vi "rio_veloster11.vi"() -> ()   [LabVIEW 2015]
uses:
  <vilib>/FPGAPlugInAG/cRIO-9113/niLvFpga_Open_cRIO-9113.vi
  <vilib>/rvi/interface/common/dynamic/niFpgaDynamicAddResources.vi
  <vilib>/FPGAPlugInAG/Dynamic/niLvFpga_Abort_Dynamic.vi
  <vilib>/FPGAPlugInAG/Dynamic/niLvFpga_Run_Dynamic.vi
  rio_Global.vi
  <vilib>/Utility/error.llb/Error Cluster From Error Code.vi
  <vilib>/rvi/errors/niLvFpgaAdjustHostInterfaceError.vi
  <vilib>/Instr/_visa.llb/VISA Configure Serial Port (Instr).vi
  <vilib>/Analysis/Matrix/Numeric/Conversions/Array To Matrix - RA2.vi
  <vilib>/Analysis/Matrix/Numeric/Multiply/Multiply - RM,RM.vi
  <vilib>/Analysis/Matrix/Numeric/Add/Add - RM,RM.vi
  <vilib>/Analysis/baseanly.llb/Real Inverse Matrix.vi
  <vilib>/Analysis/Matrix/Numeric/Subtract/Subtract - RM,RM.vi
  <vilib>/Analysis/Matrix/Numeric/Conversions/Array To Matrix - RA.vi
  <vilib>/Analysis/Matrix/Numeric/Multiply/Multiply - R,RM.vi
  <vilib>/Analysis/Matrix/Numeric/Conversions/Matrix To Array - RM.vi
  <vilib>/rvi/interface/nirviOpenFPGA/nirviOpenFPGA.xnode
  FPGA Bitfiles/autonomous_FPGATarget2_fpga4_FZHAM7r+pqE.lvbitx
  fpga/fpga4.vi
  <vilib>/rvi/interface/nirviMethod/nirviMethod.xnode
  <vilib>/rvi/interface/nirviReadWriteControl/nirviReadWriteControl.xnode
  <vilib>/Analysis/Matrix/NI_Matrix.lvlib
  <vilib>/Analysis/NI_AALBase.lvlib
  NiFpgaLv.dll
  <vilib>/rvi/interface/Simulation/niFpgaSimulationCallBeginRW.vi
panel:
  out "Heading":dbl
  out "H_GPS":dbl
  out "pos":dbl[](array[numeric])
  in  "GPS init":bool=TRUE
  out "pos_gps":dbl[](array[numeric]) format="%#_19f"
  out "dt":dbl
  out "Pos_time 10":i32
  out "battery voltage":dbl
  out "FPGA":refnum<k20>
  in  "steer limit":dbl=100.0
  in  "buzz":bool
  out "hcount":u64=1
  out "hbias":dbl
  out "vcount":u64=1
  out "vgain":dbl=1.0
  out "T PWM":u16
  out "B PWM":u16
  out "mobileye":u8[](array[numeric])
  out "timer":u32
  out "Mobileye_time 100":u32
  out "pos error":dbl
  in  "Gear Manual":i32(slide)=1 scale=-1.0..1.0
  out "map":i32=2
  out "P, R, D":i32
  out "heading error":dbl
  out "POS init":bool
  out "VS_CAN":dbl
  in  "brake":bool
  in  "Slide":dbl(slide) min=-50.0 max=50.0 step=50.0 scale=-50.0..50.0
  out "Con_time 10":i32
  out "CAN_time 10":u32
  out "ecef ref":dbl[](array[numeric])
  out "h_gps":dbl
  out "get heading":bool
  out "get position":bool
  out "rt":dbl
  out "CAN Comm Enabled":bool
  in  "SPAS Enable":bool=TRUE
  in  "file write":bool
  out "data write":refnum<file>
  out "file rw error":errorcluster
  in  "Steer input":bool=TRUE
  in  "Manual Steering angle":dbl(knob) scale=-550.0..550.0
  out "Ref vel":dbl=1.0
  in  "Manual Speed":dbl
  in  "Velocity input":bool
  out "Auto":bool
  out "Run":bool
  out "E - STOP":bool
  # "P"
  # "R"
  # "D"
  # "Manual Steering angle"
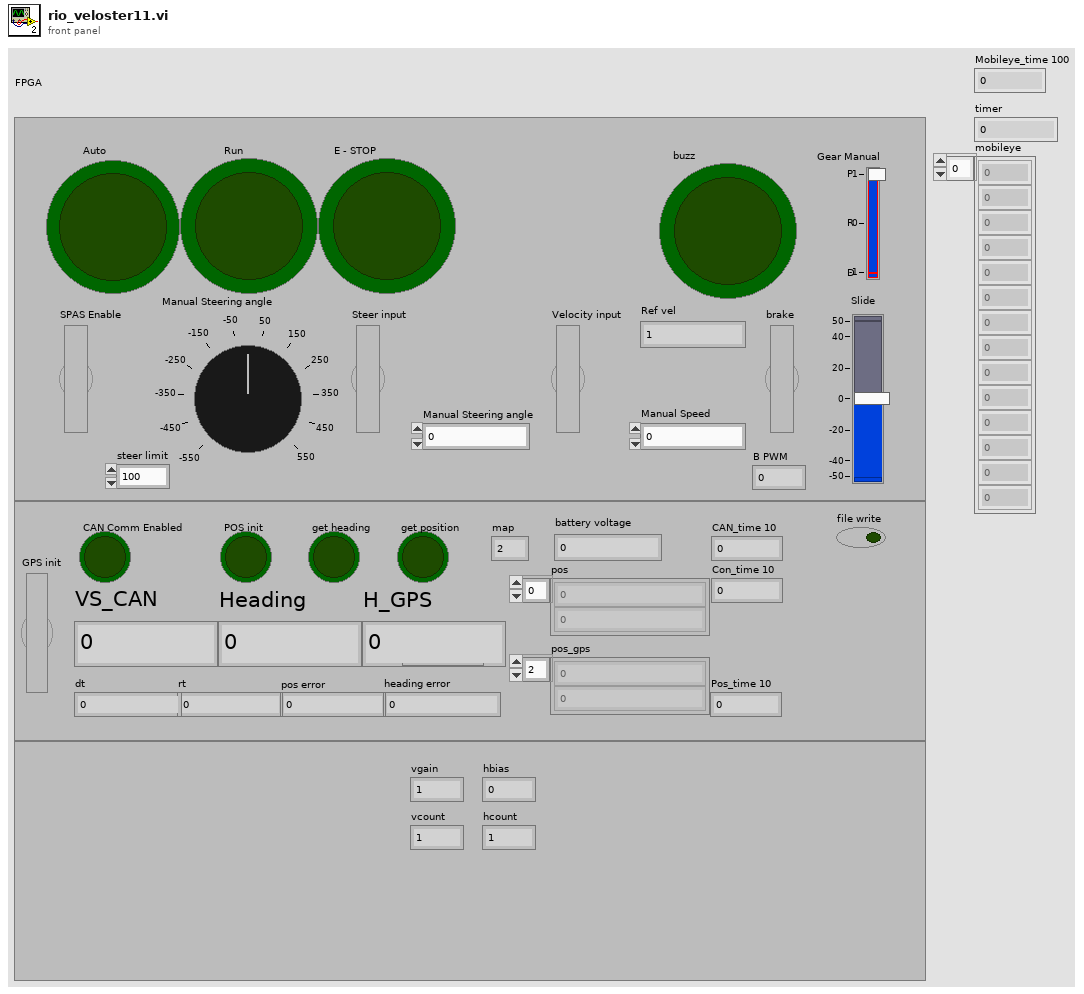
[diagram p1: front panel]
types:
  T1 = enum16{"open", "replace", "create", "open or create", "replace or create", "replace or create with confirmation"}
  T2 = cluster{"timestamp high":u32, "timestamp low":u32, "identifier":u32, "type":enum8{"Data Frame", "Remote Frame", "(reserved)", "(reserved) ", "(reserved)  ", "(reserved)   ", "Bus Error", "Transceiver Fault"}, "info A":u8, "info B":u8, "data length":u8, "data":u8[]}
  T3 = cluster{"connection ID":refnum<k16>, "net address":u32, "port":u16}
  T4 = cluster{"hash":i64, "sys time":i64, "mobileye":u8[]}
  T5 = cluster{"hash":i64, "sys time":i64, "ref_vel":dbl, "ref_steer":dbl}
  T6 = cluster{"hash":i64, "sys time":i64, "time":dbl, "yaw_rate":dbl, "mdps torque":dbl, "mdps str_ang":dbl, "VS_CAN":dbl, "lat_accel":dbl, "mcp":dbl, "accel pedal value":dbl, "tps":dbl, "odometer":dbl, "battery voltage":dbl, "WHL_SPD_RR":dbl, "WHL_SPD_RL":dbl, "WHL_SPD_FR":dbl, "WHL_SPD_FL":dbl}
  T7 = cluster{"hash":i64, "sys time":i64, "Auto":bool, "Run":bool, "Solenoid":bool, "T lim":bool, "brk_enc":u8, "B PWM":u16, "T PWM":u16, "ref_vel":dbl, "ref_bkr_enc":dbl, "ref_apv":dbl, "ref_steer":dbl}
  T8 = cluster{"hash":i64, "sys time":i64, "time":dbl, "x":dbl, "y":dbl, "h":dbl, "numSV":i32, "postype":i32, "lag":i32, "hordev":dbl, "lat":dbl, "lon":dbl, "hgt":dbl, "map_idx":i32}
  T9 = cluster{"output[0]":dbl, "output[1]":dbl, "output[2]":dbl, "output[3]":dbl, "output[4]":dbl, "output[5]":dbl, "output[6]":dbl, "output[7]":dbl, "output[8]":dbl, "output[9]":dbl, "output[10]":dbl, "output[11]":dbl, "output[12]":dbl, "output[13]":dbl, "output[14]":dbl}
  T10 = cluster{"hash":i64, "sys time":i64, "time":dbl, "speed":dbl, "heading":dbl, "lat":dbl, "lon":dbl}
  T11 = cluster{"output[0]":dbl, "output[1]":dbl, "output[2]":dbl, "output[3]":dbl, "output[4]":dbl, "output[5]":dbl, "output[6]":dbl}
  T12 = typedef "NI_Matrix.lvlib/RealMatrix.ctl" = dbl[][]
  T13 = cluster{"hash":i64, "sys time":i64, "dt":dbl, "x":dbl, "y":dbl, "speed":dbl, "heading":dbl, "yaw_rate":dbl}
  T14 = cluster{"Real 2D Array[0]":dbl, "Real 2D Array[1]":dbl, "Real 2D Array[2]":dbl, "Real 2D Array[3]":dbl, "Real 2D Array[4]":dbl}
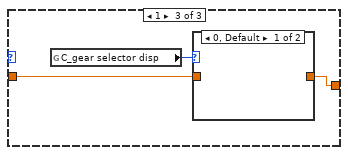
[diagram p3: hidden frame]
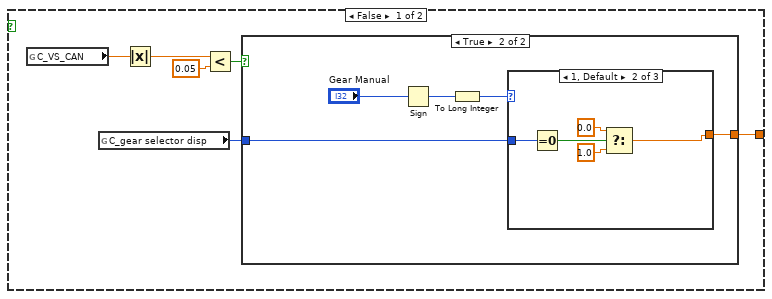
[diagram p5: hidden frame]
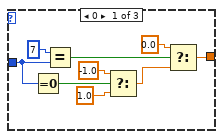
[diagram p7: hidden frame]
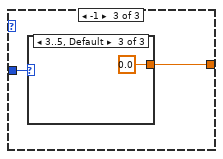
[diagram p8: hidden frame]
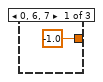
[diagram p9: hidden frame]
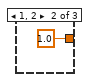
[diagram p10: hidden frame]
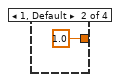
[diagram p12: hidden frame]
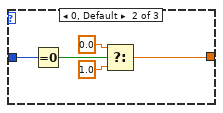
[diagram p15: hidden frame]
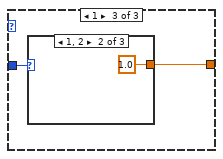
[diagram p16: hidden frame]
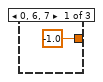
[diagram p17: hidden frame]
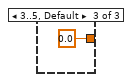
[diagram p18: hidden frame]
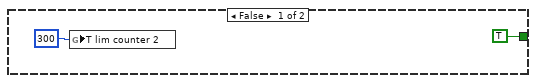
[diagram p19: hidden frame]
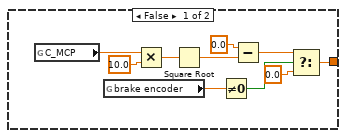
[diagram p20: hidden frame]
diagram:
  n1 = flat-sequence {
    frame #0 {
      w7 = u16 7668 ("port")
      w11 = u16 7667 ("port")
      n2 = disable-structure shown="Enabled" {
        frame Disabled {
        }
        frame Enabled {
          w21 = 0.0 ("Ref_str_ang")
          w22 = 1000.0 ("PWM GAS")
          n3 = global write "rio_Global.vi" "steering torque"(0.0 ("steering")) -> ()
          n4 = global write "rio_Global.vi" "Auto SW"(FALSE ("Auto SW")) -> ()
          n5 = global write "rio_Global.vi" "Solenoid"(FALSE ("CAN A 1")) -> ()
          n6 = global write "rio_Global.vi" "T lim counter 2"(u16 300 ("T lim counter 2")) -> ()
          n7 = global write "rio_Global.vi" "PWM GAS"(w22) -> ()
          n8 = global write "rio_Global.vi" "PWM Brake"(w22) -> ()
          n9 = global write "rio_Global.vi" "Ref_VS"(w21) -> ()
          n10 = global write "rio_Global.vi" "Ref_str_ang"(w21) -> ()
        }
      }
      n11 = xnode "Open FPGA VI Reference"() -> ("FPGA VI Reference Out"=w19:refnum<k20>, "error out"=w18:errorcluster)  [unwired: 2 in]
      n12 = global read "rio_Global.vi" "LCM PC"() -> (w3:T3)
      n13 = case shown="True" "file write" {
        frame False {
        }
        frame True {
          n14 = Open/Create/Replace File(file path (use dialog)=path "c:/datasave", operation (0:open)=T1."replace or create", access (0:read/write)=enum16{"read/write", "read-only", "write-only"}."write-only") -> (refnum out=→"data write":refnum<file>, cancelled=w29:bool, error out=→"file rw error":errorcluster)  [unwired: 3 in]
          n15 = Not(x=w29) -> (.not. x?=w28:bool)
          n16 = local write "file write"(w28) -> ()
        }
      }
      n17 = Decrement(x=w11) -> (x-1=w10:u16)
      n18 = UDP Open(11:w7) -> (port=w9:refnum<k16>)  [unwired: 4 in, 2 out]
      n19 = xnode "Invoke Method"("FPGA VI Reference In"=w19, "error in"=w18) -> ("FPGA VI Reference Out"=w17:refnum<k20>, "error out"=w16:errorcluster)
      n20 = Bundle By Name(cluster=w3, "port"=w7, "connection ID"=w9, "net address"=u32 0) -> (w4:T3)
      n21 = UDP Open(11:w10) -> (port=w13:refnum<k16>)  [unwired: 4 in, 2 out]
      n22 = xnode "Invoke Method"("FPGA VI Reference In"=w17, "error in"=w16, "Wait Until Done (F)"=FALSE) -> ("FPGA VI Reference Out"=→"FPGA":refnum<k20>)  [unwired: 1 out]
      n23 = global read "rio_Global.vi" "LCM"() -> (w6:T3)
      n24 = global write "rio_Global.vi" "LCM PC"(w4) -> ()
      n25 = Bundle By Name(cluster=w6, "port"=w11, "connection ID"=w13, "net address"=u32 4294967295) -> (w5:T3)
      n26 = global write "rio_Global.vi" "LCM"(w5) -> ()
    }
    frame #1 {
      n27 = disable-structure shown="Enabled" {
        frame Enabled {
          n28 = while {
            stop <- FALSE stop-if-true
            n29 = flat-sequence {
              frame #0 {
                n30 = Wait Until Next ms Multiple(millisecond multiple=u32 100) -> (millisecond timer value=w141:u32)
                n31 = feedback #1(w141) -> (w139:u32)
                n32 = feedback-in #1(w141) -> ()
                n33 = Subtract(x=w141, y=w139) -> (x-y=→"Mobileye_time 100":u32)
              }
              frame #1 {
                n34 = local read "FPGA"() -> (w187:refnum<k20>)
                n35 = xnode "Read/Write Control"("FPGA VI Reference In"=w187) -> ("m 700"=w147:u8[], "m 760"=w183:u8[], "m 710"=w172:u8[], "m 711"=w168:u8[], "m 720"=w166:u8[], "m 721"=w165:u8[], "m 722"=w164:u8[], "m 723"=w163:u8[], "m 724"=w162:u8[], "m 725"=w161:u8[], "m 726"=w160:u8[], "m 727"=w159:u8[], "m 728"=w158:u8[], "m 729"=w157:u8[])  [unwired: 1 in, 2 out]
                n36 = Build Array(w166, w165, w164, w163, w162, w161, w160, w159, w158, w157) -> (w156:u8[][])
                n37 = Array Subset(array=w147, index=0, length=4) -> (w144:u8[])
                n38 = Array Subset(array=w168, index=6, length=6) -> (w167:u8[])
                n39 = Index Array(array=w147, index #1=4 ("index"), index #4=8 ("index"), index #5=11 ("index")) -> (element #1=w180:u8, element #2=w179:u8, element #3=w178:u8, element #4=w177:u8, element #5=w176:u8)  [unwired: 2 in]
                n40 = Index Array(array=w144, index #1=0 ("index")) -> (element #1=w153:u8, element #2=w152:u8, element #3=w151:u8, element #4=w150:u8)  [unwired: 3 in]
                n41 = Array Subset(array=w183, index=4, length=3) -> (w175:u8[])
                n42 = Array Subset(array=w172, index=5, length=7) -> (w171:u8[])
                n43 = Build Array (concatenate)(w144, w180, w179, w178, w177, w176, w175, w171, w167) -> (w155:u8[])
                n44 = Join Numbers(hi=w153, lo=w152) -> ((hi.lo)=w149:u16)
                n45 = Join Numbers(hi=w151, lo=w150) -> ((hi.lo)=w148:u16)
                n46 = for {
                  tunnel: w156 -> [w189] mode=indexing
                  shift-right: [w192] -> w142
                  shift-left: w155 -> [w193]
                  n47 = Array Subset(array=w189, index=4, length=8) -> (w188:u8[])
                  n48 = disable-structure shown="Enabled" {
                    disable-tunnel: [w196 TRUE ("lsb carry out")] -> w194
                    disable-tunnel: w188 -> [w195 _]
                    frame Disabled {
                      n49 = Index Array(array=w195, index=0) -> (element=w198:u8)
                      n50 = Rotate Right With Carry(2:w198, 3:FALSE ("carry")) -> (1:w196:bool)  [unwired: 1 out]
                    }
                    frame Enabled {
                    }
                  }
                  n51 = case shown="True" w194 {
                    tunnel: w193 -> [w201 w204]
                    tunnel: [w201 w203] -> w192
                    tunnel: w188 -> [_ w202]
                    frame False {
                    }
                    frame True {
                      n52 = Build Array (concatenate)(w204, w202) -> (w203:u8[])
                    }
                  }
                }
                "mobileye" <- w142
                n53 = Join Numbers(hi=w149, lo=w148) -> ((hi.lo)=→"timer":u32)
              }
              frame #2 {
                n54 = Get Date/Time In Seconds() -> (seconds since 1Jan1904=w211:timestamp)
                n55 = To Double Precision Float(number=w211) -> (double precision float=w210:dbl)
                n56 = global read "rio_Global.vi" "LCM_EYE_RAW_T"() -> (w205:T4)
                n57 = Unbundle By Name(w205) -> ("hash"=w218:i64)
                n58 = Multiply(x=w210, y=1000000.0) -> (x*y=w208:dbl)
                n59 = local read "mobileye"() -> (w212:u8[])
                n60 = call "hash.vi"("input"=w218) -> ("output"=w217:i64)  [unwired: 10 in]
                n61 = To Quad Integer(1:w208) -> (0:w207:i64)
                n62 = Bundle By Name(cluster=w205, "hash"=w217, "sys time"=w207, "mobileye"=w212) -> (w216:T4)
                n63 = Flatten To String(anything=w216, prepend array or string size? (T)=FALSE) -> (data string=w215:string)  [unwired: 2 in, 2 out]
                n64 = global read "rio_Global.vi" "LCM"() -> (w206:T3)
                n65 = call "LCM_send.vi"("DATA"=w215, "ID"="EYE_RAW_T", "LCM"=w206) -> ()  [unwired: 6 in, 3 out]
              }
            }
          }
        }
        frame Disabled {
        }
      }
      n66 = while {
        stop <- FALSE stop-if-true
        n67 = global read "rio_Global.vi" "LCM PC"() -> (w128:T3)
        n68 = call "LCM_read.vi"("LCM"=w128) -> ("data"=w126:string, "ID"=w127:string)  [unwired: 7 in, 2 out]
        n69 = case shown="\"CON_INPUT_T\"" w127 {
          tunnel: w126 -> [_ w129]
          frame "False", Default {
          }
          frame "CON_INPUT_T" {
            n70 = global read "rio_Global.vi" "CON_INPUT_T"() -> (w131:T5)
            n71 = Unflatten From String(type=w131, binary string=w129, data includes array or string size? (T)=FALSE) -> (value=w130:T5, error out=w132:errorcluster)  [unwired: 2 in, 1 out]
            n72 = case shown="No Error" w132 {
              tunnel: w130 -> [w136 _]
              frame No Error {
                n73 = Unbundle By Name(w136) -> ("ref_vel"=w135:dbl, "ref_steer"=w134:dbl)
                n74 = global write "rio_Global.vi" "Ref_VS"(w135) -> ()
                n75 = global write "rio_Global.vi" "Ref_str_ang"(w134) -> ()
              }
              frame Error {
              }
            }
          }
        }
      }
      n76 = while {
        stop <- FALSE stop-if-true
        n77 = flat-sequence {
          tunnel: [w40] -> w34
          tunnel: w34 -> [w57]
          tunnel: [w56] -> w33
          tunnel: w33 -> [w111]
          frame #0 {
            n78 = Wait Until Next ms Multiple(millisecond multiple=u32 10) -> ()  [unwired: 1 out]
          }
          frame #1 {
            n79 = local read "FPGA"() -> (w42:refnum<k20>)
            n80 = xnode "Read/Write Control"("FPGA VI Reference In"=w42) -> ("FPGA VI Reference Out"=w40:refnum<k20>, "Auto"=w41:bool, "Run"=w43:bool, "T Lim"=w37:bool, "brk enc"=w53:u8)  [unwired: 1 in, 1 out]
            "Auto" <- w41
            n81 = global write "rio_Global.vi" "Auto"(w41) -> ()
            n82 = global write "rio_Global.vi" "T Lim"(w37) -> ()
            n83 = To Double Precision Float(number=w53) -> (double precision float=w45:dbl)
            n84 = And(x=w41, y=w43) -> (x .and. y?=w38:bool)
            "Run" <- w38
            n85 = global write "rio_Global.vi" "Run"(w38) -> ()
            n86 = Subtract(x=w45, y=220.0) -> (x-y=w47:dbl)
            n87 = Not(x=w38) -> (.not. x?=w55:bool)
            n88 = Multiply(x=w47, y=-100.0) -> (x*y=w50:dbl)
            n89 = And(x=w41, y=w55) -> (x .and. y?=→"E - STOP":bool)
            n90 = Divide(x=w50, y=175.0) -> (x/y=w51:dbl)
            n91 = In Range and Coerce(upper limit=100.0, x=w51, lower limit=0.0) -> (coerced(x)=w39:dbl)  [unwired: 1 out]
            n92 = global write "rio_Global.vi" "brake encoder"(w39) -> ()
          }
          frame #2 {
            n93 = global read "rio_Global.vi" "steering angle"() -> (w80:dbl)
            n94 = Multiply(x=w80, y=10.0) -> (x*y=w62:dbl)
            n95 = Greater Than 0?(x=w62) -> (x > 0?=w61:bool)
            n96 = Add(x=w62, y=65536.0) -> (x+y=w64:dbl)
            n97 = Select(t=w62, s=w61, f=w64) -> (s? t:f=w65:dbl)
            n98 = To Unsigned Word Integer(number=w65) -> (unsigned 16bit integer=w66:u16)
            n99 = Split Number(x=w66) -> (hi(x)=w67:u8, lo(x)=w68:u8)
            n100 = feedback #2(u8 0 ("Con steer alivecnt")) -> (w77:u8)
            n101 = Increment(x=w77) -> (x+1=w76:u8)
            n102 = feedback-in #2(w76) -> ()
            n103 = Build Array(u8 0 ("Con steer status"), w68, w67, u8 0 ("element"), w77, u8 0 ("element"), u8 0 ("element")) -> (w73:u8[])
            n104 = global read "rio_Global.vi" "Auto"() -> (w79:bool)
            n105 = Add Array Elements(numeric array=w73) -> (sum=w72:u8)
            n106 = And(x=w79, y="SPAS Enable") -> (x .and. y?=w58:bool)
            n107 = Build Array (concatenate)(w73, w72) -> (w78:u8[])
            n108 = case shown="True" w58 {
              tunnel: w78 -> [_ w86]
              tunnel: w57 -> [w82 w85]
              tunnel: [w81 w84] -> w56
              frame False {
                n109 = xnode "Read/Write Control"("FPGA VI Reference In"=w82, "send can"=FALSE) -> ("FPGA VI Reference Out"=w81:refnum<k20>)  [unwired: 1 in, 1 out]
              }
              frame True {
                n110 = disable-structure shown="Enabled" {
                  disable-tunnel: w86 -> [w92 _]
                  disable-tunnel: w85 -> [w88 w110]
                  disable-tunnel: [w87 w110] -> w84
                  frame Enabled {
                    n111 = flat-sequence {
                      tunnel: w92 -> [w96]
                      tunnel: [w96] -> w91
                      tunnel: [w94] -> w90
                      tunnel: w88 -> [w93]
                      tunnel: w91 -> [w101]
                      tunnel: w90 -> [w99]
                      tunnel: [w98] -> w89
                      tunnel: w89 -> [w105]
                      tunnel: [w104] -> w87
                      frame #0 {
                        n112 = xnode "Read/Write Control"("FPGA VI Reference In"=w93, "send can"=TRUE) -> ("FPGA VI Reference Out"=w94:refnum<k20>)  [unwired: 1 in, 1 out]
                      }
                      frame #1 {
                        n113 = Bundle By Name(cluster=T2 {"timestamp high"=0, "timestamp low"=0, "identifier"=0, "type"=enum."Data Frame", "info A"=0, "info B"=0, "data length"=8, "data"=[0, 0, 0, 0, 0, 0, 0, 0]} ("Mod4/CAN1 input"), "identifier"=u32 912, "data"=w101, "data length"=u8 8) -> (w100:T2)
                        n114 = xnode "Read/Write Control"("FPGA VI Reference In"=w99, "Mod4/CAN1 input"=w100) -> ("FPGA VI Reference Out"=w98:refnum<k20>)  [unwired: 1 in, 1 out]
                      }
                      frame #2 {
                        n115 = disable-structure shown="Enabled" {
                          disable-tunnel: w105 -> [w108 w109]
                          disable-tunnel: [w106 w109] -> w104
                          frame Disabled {
                            n116 = xnode "Read/Write Control"("FPGA VI Reference In"=w108, "send can"=FALSE) -> ("FPGA VI Reference Out"=w106:refnum<k20>)  [unwired: 1 in, 1 out]
                          }
                          frame Enabled {
                          }
                        }
                      }
                    }
                  }
                  frame Disabled {
                  }
                }
              }
            }
          }
          frame #3 {
            n117 = disable-structure shown="Enabled" {
              disable-tunnel: [w122 _] -> w116
              frame Enabled {
                n118 = global read "rio_Global.vi" "Auto"() -> (w121:bool)
                n119 = global read "rio_Global.vi" "Run"() -> (w120:bool)
                n120 = Compound Arithmetic op=AND(w121, w120) -> (w124:bool)
                n121 = And(x=w124, y="buzz") -> (x .and. y?=w122:bool)
              }
              frame Disabled {
              }
            }
            n122 = global read "rio_Global.vi" "PWM Brake"() -> (w114:dbl)
            n123 = global read "rio_Global.vi" "PWM GAS"() -> (w113:dbl)
            n124 = global read "rio_Global.vi" "PWM Shift"() -> (w119:dbl)
            n125 = To Unsigned Word Integer(number=w114) -> (unsigned 16bit integer=w118:u16)
            "B PWM" <- w118
            n126 = To Unsigned Word Integer(number=w113) -> (unsigned 16bit integer=w115:u16)
            "T PWM" <- w115
            n127 = global read "rio_Global.vi" "Solenoid"() -> (w112:bool)
            n128 = To Unsigned Word Integer(number=w119) -> (unsigned 16bit integer=w117:u16)
            n129 = xnode "Read/Write Control"("FPGA VI Reference In"=w111, "Buzz"=w116, "S Pwm 1"=w117, "S Pwm 2"=w117, "B Pwm"=w118, "T Pwm"=w115, "Solenoid"=w112) -> ()  [unwired: 1 in, 2 out]
          }
        }
      }
      n130 = while {
        stop <- FALSE stop-if-true
        n131 = flat-sequence {
          frame #0 {
            n132 = Wait Until Next ms Multiple(millisecond multiple=u32 10) -> (millisecond timer value=w222:u32)
            n133 = feedback #3(w222) -> (w221:u32)
            n134 = feedback-in #3(w222) -> ()
            n135 = Subtract(x=w222, y=w221) -> (x-y=→"CAN_time 10":u32)
          }
          frame #1 {
            n136 = disable-structure shown="Enabled" {
              disable-tunnel: [w225 _] -> w224
              frame Enabled {
                n137 = for {
                  tunnel: u32[] [356, 544, 809, 914, 1087, 1200, 1264, 1349] -> [w229] mode=indexing
                  tunnel: [w228] -> w226 mode=indexing
                  n138 = case shown="43F" w229 {
                    tunnel: [_ w230 w305 w344 w403 w427 w498 w530] -> w228
                    frame 0, Default {
                    }
                    frame 544 {
                      n139 = flat-sequence {
                        tunnel: [w237] -> w230
                        tunnel: [w236] -> w231
                        frame #0 {
                          n140 = local read "FPGA"() -> (w242:refnum<k20>)
                          n141 = xnode "Read/Write Control"("FPGA VI Reference In"=w242) -> ("can 220"=w241:u8[])  [unwired: 1 in, 2 out]
                          n142 = Index Array(array=w241, index #1=0 ("index")) -> (element #1=w248:u8, element #2=w247:u8, element #3=w246:u8, element #4=w245:u8)  [unwired: 3 in]
                          n143 = Join Numbers(hi=w248, lo=w247) -> ((hi.lo)=w244:u16)
                          n144 = Join Numbers(hi=w246, lo=w245) -> ((hi.lo)=w243:u16)
                          n145 = Join Numbers(hi=w244, lo=w243) -> ((hi.lo)=w234:u32)
                          n146 = Array Subset(array=w241, index=4) -> (w236:u8[])  [unwired: 1 in]
                          n147 = global write "rio_Global.vi" "C_time"(w234) -> ()
                          n148 = feedback #4(u32 0) -> (w238:u32)
                          n149 = feedback-in #4(w234) -> ()
                          n150 = Multiply(x=w234, y=1e-07) -> (x*y=w232:dbl)
                          n151 = Not Equal?(x=w234, y=w238) -> (x != y?=w237:bool)
                          n152 = feedback-in #5(w232) -> ()
                          n153 = feedback #5(w232) -> (w233:dbl)
                          n154 = global write "rio_Global.vi" "C_ts"(w233) -> ()
                        }
                      }
                      n155 = case shown="True" w230 {
                        tunnel: w231 -> [_ w283]
                        frame False {
                        }
                        frame True {
                          w253 = u16 8191
                          w260 = u16 2047
                          n156 = Index Array(array=w283, index #1=5 ("index"), index #2=4 ("index"), index #3=1 ("index"), index #4=0 ("index"), index #5=7 ("index"), index #6=6 ("index")) -> (element #1=w276:u8, element #2=w275:u8, element #3=w274:u8, element #4=w273:u8, element #5=w272:u8, element #6=w271:u8)
                          n157 = Join Numbers(hi=w274, lo=w273) -> ((hi.lo)=w261:u16)
                          n158 = Join Numbers(hi=w272, lo=w271) -> ((hi.lo)=w252:u16)
                          n159 = And(x=w276, y=u8 15) -> (x .and. y?=w269:u8)
                          n160 = Logical Shift(y=i16 -6, x=w274) -> (x << y=w263:u8)
                          n161 = Logical Shift(y=i16 -6, x=w272) -> (x << y=w256:u8)
                          n162 = Join Numbers(hi=w269, lo=w275) -> ((hi.lo)=w266:u16)
                          n163 = Equal To 0?(x=w263) -> (x = 0?=w264:bool)
                          n164 = And(x=w260, y=w261) -> (x .and. y?=w259:u16)
                          n165 = And(x=w253, y=w252) -> (x .and. y?=w251:u16)
                          n166 = Not Equal?(x=w260, y=w259) -> (x != y?=w265:bool)
                          n167 = Not Equal?(x=w253, y=w251) -> (x != y?=w254:bool)
                          n168 = Equal To 0?(x=w256) -> (x = 0?=w255:bool)
                          n169 = Not Equal?(x=u16 4095, y=w266) -> (x != y?=w267:bool)
                          n170 = case shown="True" w267 {
                            tunnel: w266 -> [_ w303]
                            frame False {
                            }
                            frame True {
                              n171 = global write "rio_Global.vi" "C_MCP"(w303) -> ()
                              n172 = Greater?(x=w303, y=u16 10) -> (0:w302:bool)
                              n173 = global write "rio_Global.vi" "C_Brake"(w302) -> ()
                            }
                          }
                          n174 = And(x=w264, y=w265) -> (x .and. y?=w258:bool)
                          n175 = And(x=w255, y=w254) -> (x .and. y?=w250:bool)
                          n176 = case shown="True" w258 {
                            tunnel: w259 -> [_ w301]
                            frame False {
                            }
                            frame True {
                              n177 = To Double Precision Float(number=w301) -> (double precision float=w300:dbl)
                              n178 = Multiply(x=w300, y=0.01) -> (x*y=w298:dbl)
                              n179 = Subtract(x=w298, y=10.23) -> (x-y=w296:dbl)
                              n180 = global write "rio_Global.vi" "C_lat_accel"(w296) -> ()
                            }
                          }
                          n181 = case shown="True" w250 {
                            tunnel: w251 -> [_ w295]
                            frame False {
                            }
                            frame True {
                              n182 = To Double Precision Float(number=w295) -> (double precision float=w294:dbl)
                              n183 = Multiply(x=w294, y=0.01) -> (x*y=w292:dbl)
                              n184 = Subtract(x=w292, y=40.95) -> (x-y=w286:dbl)
                              n185 = Add(x=w286, y=-0.034) -> (x+y=w285:dbl)
                              n186 = Multiply(x=w285, y=1.045) -> (x*y=w288:dbl)
                              n187 = Add(x=w288, y=0.0) -> (x+y=w284:dbl)
                              n188 = global write "rio_Global.vi" "C_yaw_rate"(w284) -> ()
                            }
                          }
                        }
                      }
                    }
                    frame 809 {
                      n189 = flat-sequence {
                        tunnel: [w308] -> w305
                        tunnel: [w307] -> w306
                        frame #0 {
                          n190 = local read "FPGA"() -> (w314:refnum<k20>)
                          n191 = xnode "Read/Write Control"("FPGA VI Reference In"=w314) -> ("can 329"=w313:u8[])  [unwired: 1 in, 2 out]
                          n192 = Index Array(array=w313, index #1=0 ("index")) -> (element #1=w320:u8, element #2=w319:u8, element #3=w318:u8, element #4=w317:u8)  [unwired: 3 in]
                          n193 = Join Numbers(hi=w320, lo=w319) -> ((hi.lo)=w316:u16)
                          n194 = Join Numbers(hi=w318, lo=w317) -> ((hi.lo)=w315:u16)
                          n195 = Join Numbers(hi=w316, lo=w315) -> ((hi.lo)=w309:u32)
                          n196 = Array Subset(array=w313, index=4) -> (w307:u8[])  [unwired: 1 in]
                          n197 = feedback #6(u32 0) -> (w310:u32)
                          n198 = feedback-in #6(w309) -> ()
                          n199 = Not Equal?(x=w309, y=w310) -> (x != y?=w308:bool)
                        }
                      }
                      n200 = case shown="True" w305 {
                        tunnel: w306 -> [_ w331]
                        frame False {
                        }
                        frame True {
                          # "10ms"
                          n201 = Index Array(array=w331, index #1=5 ("index"), index #2=6 ("index"), index #3=4 ("index")) -> (element #1=w328:u8, element #2=w325:u8)  [unwired: 1 out]
                          n202 = Not Equal?(x=w328, y=u8 255 ("x")) -> (x != y?=w324:bool)
                          n203 = Not Equal?(x=w325, y=u8 255 ("x")) -> (x != y?=w323:bool)
                          n204 = case shown="True" w324 {
                            tunnel: w328 -> [_ w343]
                            frame False {
                            }
                            frame True {
                              n205 = Subtract(x=w343, y=u8 32) -> (x-y=w341:u8)
                              n206 = To Double Precision Float(number=w341) -> (double precision float=w340:dbl)
                              n207 = Multiply(x=w340, y=100.0) -> (x*y=w338:dbl)
                              n208 = Divide(x=w338, y=213.0) -> (x/y=w336:dbl)
                              n209 = global write "rio_Global.vi" "C_tps"(w336) -> ()
                            }
                          }
                          n210 = case shown="True" w323 {
                            tunnel: w325 -> [_ w335]
                            frame False {
                            }
                            frame True {
                              n211 = To Double Precision Float(number=w335) -> (double precision float=w334:dbl)
                              n212 = Multiply(x=w334, y=0.3906) -> (x*y=w332:dbl)
                              n213 = global write "rio_Global.vi" "C_APV"(w332) -> ()
                            }
                          }
                        }
                      }
                    }
                    frame 914 {
                      n214 = flat-sequence {
                        tunnel: [w347] -> w344
                        tunnel: [w346] -> w345
                        frame #0 {
                          n215 = local read "FPGA"() -> (w353:refnum<k20>)
                          n216 = xnode "Read/Write Control"("FPGA VI Reference In"=w353) -> ("can 392"=w352:u8[])  [unwired: 1 in, 2 out]
                          n217 = Index Array(array=w352, index #1=0 ("index")) -> (element #1=w359:u8, element #2=w358:u8, element #3=w357:u8, element #4=w356:u8)  [unwired: 3 in]
                          n218 = Join Numbers(hi=w359, lo=w358) -> ((hi.lo)=w355:u16)
                          n219 = Join Numbers(hi=w357, lo=w356) -> ((hi.lo)=w354:u16)
                          n220 = Join Numbers(hi=w355, lo=w354) -> ((hi.lo)=w348:u32)
                          n221 = Array Subset(array=w352, index=4) -> (w346:u8[])  [unwired: 1 in]
                          n222 = feedback #7(u32 0) -> (w349:u32)
                          n223 = feedback-in #7(w348) -> ()
                          n224 = Not Equal?(x=w348, y=w349) -> (x != y?=w347:bool)
                        }
                      }
                      n225 = case shown="True" w344 {
                        tunnel: w345 -> [_ w367]
                        frame False {
                        }
                        frame True {
                          # "20ms"
                          n226 = Array Subset(array=w367, index=0, length=7) -> (w364:u8[])
                          n227 = Index Array(array=w367, index #1=7 ("index"), index #2=2 ("index"), index #3=1 ("index"), index #4=4 ("index"), index #5=3 ("index")) -> (element #1=w361:u8, element #2=w373:u8, element #3=w372:u8, element #4=w369:u8, element #5=w368:u8)
                          n228 = Add Array Elements(numeric array=w364) -> (sum=w362:u8)
                          n229 = Equal?(x=w362, y=w361) -> (x = y?=w363:bool)
                          n230 = case shown="True" w363 {
                            tunnel: w373 -> [_ w387]
                            tunnel: w372 -> [_ w386]
                            tunnel: w369 -> [_ w383]
                            tunnel: w368 -> [_ w382]
                            frame False {
                            }
                            frame True {
                              w378 = u16 4095 ("y")
                              n231 = Join Numbers(hi=w387, lo=w386) -> ((hi.lo)=w379:u16)
                              n232 = Join Numbers(hi=w383, lo=w382) -> ((hi.lo)=w384:u16)
                              n233 = And(x=w378, y=w379) -> (x .and. y?=w377:u16)
                              n234 = Not Equal?(x=w384, y=u16 32767 ("x")) -> (x != y?=w380:bool)
                              n235 = Not Equal?(x=w378, y=w377) -> (x != y?=w381:bool)
                              n236 = case shown="True" w381 {
                                tunnel: w377 -> [_ w400]
                                frame False {
                                }
                                frame True {
                                n237 = To Double Precision Float(number=w400) -> (double precision float=w399:dbl)
                                n238 = Subtract(x=w399, y=2048.0) -> (x-y=w398:dbl)
                                n239 = Multiply(x=w398, y=0.01) -> (x*y=w397:dbl)
                                n240 = global write "rio_Global.vi" "C_mdps torque"(w397) -> ()
                                }
                              }
                              n241 = case shown="True" w380 {
                                tunnel: w384 -> [_ w394]
                                frame False {
                                }
                                frame True {
                                n242 = To Double Precision Float(number=w394) -> (double precision float=w391:dbl)
                                n243 = Subtract(x=w391, y=65536.0) -> (x-y=w392:dbl)
                                n244 = Greater?(x=w391, y=32767.0 ("x")) -> (0:w395:bool)
                                n245 = Select(t=w392, s=w395, f=w391) -> (s? t:f=w390:dbl)
                                n246 = Multiply(x=w390, y=0.1) -> (x*y=w388:dbl)
                                n247 = global write "rio_Global.vi" "C_mdps str_ang"(w388) -> ()
                                }
                              }
                            }
                          }
                        }
                      }
                    }
                    frame 1087 {
                      n248 = flat-sequence {
                        tunnel: [w406] -> w403
                        tunnel: [w405] -> w404
                        frame #0 {
                          n249 = local read "FPGA"() -> (w412:refnum<k20>)
                          n250 = xnode "Read/Write Control"("FPGA VI Reference In"=w412) -> ("can 43F"=w411:u8[])  [unwired: 1 in, 2 out]
                          n251 = Index Array(array=w411, index #1=0 ("index")) -> (element #1=w418:u8, element #2=w417:u8, element #3=w416:u8, element #4=w415:u8)  [unwired: 3 in]
                          n252 = Join Numbers(hi=w418, lo=w417) -> ((hi.lo)=w414:u16)
                          n253 = Join Numbers(hi=w416, lo=w415) -> ((hi.lo)=w413:u16)
                          n254 = Join Numbers(hi=w414, lo=w413) -> ((hi.lo)=w407:u32)
                          n255 = Array Subset(array=w411, index=4) -> (w405:u8[])  [unwired: 1 in]
                          n256 = feedback #8(u32 0) -> (w408:u32)
                          n257 = feedback-in #8(w407) -> ()
                          n258 = Not Equal?(x=w407, y=w408) -> (x != y?=w406:bool)
                        }
                      }
                      n259 = case shown="True" w403 {
                        tunnel: w404 -> [_ w425]
                        frame False {
                        }
                        frame True {
                          w422 = u8 15 ("y")
                          # "10ms"
                          n260 = Index Array(array=w425, index=1) -> (element=w423:u8)
                          n261 = And(x=w423, y=w422) -> (x .and. y?=w421:u8)
                          n262 = Not Equal?(x=w421, y=w422) -> (x != y?=w420:bool)
                          n263 = case shown="True" w420 {
                            tunnel: w421 -> [_ w426]
                            frame False {
                            }
                            frame True {
                              n264 = global write "rio_Global.vi" "C_gear selector disp"(w426) -> ()
                            }
                          }
                        }
                      }
                    }
                    frame 1200 {
                      n265 = flat-sequence {
                        tunnel: [w430] -> w427
                        tunnel: [w429] -> w428
                        frame #0 {
                          n266 = local read "FPGA"() -> (w436:refnum<k20>)
                          n267 = xnode "Read/Write Control"("FPGA VI Reference In"=w436) -> ("can 4B0"=w435:u8[])  [unwired: 1 in, 2 out]
                          n268 = Index Array(array=w435, index #1=0 ("index")) -> (element #1=w442:u8, element #2=w441:u8, element #3=w440:u8, element #4=w439:u8)  [unwired: 3 in]
                          n269 = Join Numbers(hi=w442, lo=w441) -> ((hi.lo)=w438:u16)
                          n270 = Join Numbers(hi=w440, lo=w439) -> ((hi.lo)=w437:u16)
                          n271 = Join Numbers(hi=w438, lo=w437) -> ((hi.lo)=w431:u32)
                          n272 = Array Subset(array=w435, index=4) -> (w429:u8[])  [unwired: 1 in]
                          n273 = feedback #9(u32 0) -> (w432:u32)
                          n274 = feedback-in #9(w431) -> ()
                          n275 = Not Equal?(x=w431, y=w432) -> (x != y?=w430:bool)
                        }
                      }
                      n276 = case shown="True" w427 {
                        tunnel: w428 -> [_ w473]
                        frame False {
                        }
                        frame True {
                          w447 = u16 16383 ("x")
                          w460 = u16 16383 ("x")
                          # "20ms"
                          n277 = Index Array(array=w473, index #1=1 ("index"), index #2=0 ("index"), index #3=3 ("index"), index #4=2 ("index"), index #5=5 ("index"), index #6=4 ("index"), index #7=7 ("index"), index #8=6 ("index")) -> (element #1=w452:u8, element #2=w451:u8, element #3=w450:u8, element #4=w449:u8, element #5=w470:u8, element #6=w469:u8, element #7=w465:u8, element #8=w464:u8)
                          n278 = Join Numbers(hi=w452, lo=w451) -> ((hi.lo)=w448:u16)
                          n279 = Join Numbers(hi=w450, lo=w449) -> ((hi.lo)=w446:u16)
                          n280 = Join Numbers(hi=w470, lo=w469) -> ((hi.lo)=w468:u16)
                          n281 = Join Numbers(hi=w465, lo=w464) -> ((hi.lo)=w461:u16)
                          n282 = And(x=w448, y=w447) -> (x .and. y?=w445:u16)
                          n283 = And(x=w447, y=w446) -> (x .and. y?=w444:u16)
                          n284 = And(x=w468, y=w460) -> (x .and. y?=w459:u16)
                          n285 = And(x=w460, y=w461) -> (x .and. y?=w458:u16)
                          n286 = Not Equal?(x=w459, y=w460) -> (x != y?=w463:bool)
                          n287 = Not Equal?(x=w460, y=w458) -> (x != y?=w462:bool)
                          n288 = And(x=w463, y=w462) -> (x .and. y?=w457:bool)
                          n289 = case shown="True" w457 {
                            tunnel: w459 -> [_ w497]
                            tunnel: w458 -> [_ w496]
                            tunnel: w445 -> [_ w490]
                            tunnel: w444 -> [_ w489]
                            frame False {
                            }
                            frame True {
                              w486 = 0.03125 ("y")
                              w495 = 0.03125 ("y")
                              n290 = To Double Precision Float(number=w490) -> (double precision float=w487:dbl)
                              n291 = To Double Precision Float(number=w489) -> (double precision float=w485:dbl)
                              n292 = To Double Precision Float(number=w497) -> (double precision float=w488:dbl)
                              n293 = To Double Precision Float(number=w496) -> (double precision float=w484:dbl)
                              n294 = Multiply(x=w487, y=w486) -> (x*y=w483:dbl)
                              n295 = Multiply(x=w486, y=w485) -> (x*y=w482:dbl)
                              n296 = Multiply(x=w488, y=w495) -> (x*y=w481:dbl)
                              n297 = Multiply(x=w495, y=w484) -> (x*y=w480:dbl)
                              n298 = global write "rio_Global.vi" "C_WHL_SPD_FL"(w483) -> ()
                              n299 = global write "rio_Global.vi" "C_WHL_SPD_FR"(w482) -> ()
                              n300 = global write "rio_Global.vi" "C_WHL_SPD_RL"(w481) -> ()
                              n301 = global write "rio_Global.vi" "C_WHL_SPD_RR"(w480) -> ()
                              n302 = Add(x=w481, y=w480) -> (x+y=w494:dbl)
                              n303 = Multiply(x=w494, y=0.5) -> (x*y=w491:dbl)
                              n304 = global read "rio_Global.vi" "C_gear selector disp"() -> (w478:u8)
                              n305 = Multiply(x=w491, y=1.028) -> (x*y=w476:dbl)
                              n306 = Negate(x=w476) -> (-x=w477:dbl)
                              n307 = Equal?(x=w478, y=u8 7) -> (x = y?=w475:bool)
                              n308 = Select(t=w477, s=w475, f=w476) -> (s? t:f=w474:dbl)
                              n309 = global write "rio_Global.vi" "C_VS_CAN"(w474) -> ()
                            }
                          }
                        }
                      }
                    }
                    frame 1264 {
                      n310 = flat-sequence {
                        tunnel: [w501] -> w498
                        tunnel: [w500] -> w499
                        frame #0 {
                          n311 = local read "FPGA"() -> (w507:refnum<k20>)
                          n312 = xnode "Read/Write Control"("FPGA VI Reference In"=w507) -> ("can 4F0"=w506:u8[])  [unwired: 1 in, 2 out]
                          n313 = Index Array(array=w506, index #1=0 ("index")) -> (element #1=w513:u8, element #2=w512:u8, element #3=w511:u8, element #4=w510:u8)  [unwired: 3 in]
                          n314 = Join Numbers(hi=w513, lo=w512) -> ((hi.lo)=w509:u16)
                          n315 = Join Numbers(hi=w511, lo=w510) -> ((hi.lo)=w508:u16)
                          n316 = Join Numbers(hi=w509, lo=w508) -> ((hi.lo)=w502:u32)
                          n317 = Array Subset(array=w506, index=4) -> (w500:u8[])  [unwired: 1 in]
                          n318 = feedback #10(u32 0) -> (w503:u32)
                          n319 = feedback-in #10(w502) -> ()
                          n320 = Not Equal?(x=w502, y=w503) -> (x != y?=w501:bool)
                        }
                      }
                      n321 = case shown="True" w498 {
                        tunnel: w499 -> [_ w527]
                        frame False {
                        }
                        frame True {
                          # "20 ms"
                          n322 = Index Array(array=w527, index #1=7 ("index"), index #2=6 ("index"), index #3=5 ("index")) -> (element #1=w521:u8, element #2=w523:u8, element #3=w522:u8)
                          n323 = Join Numbers(hi=w523, lo=w522) -> ((hi.lo)=w518:u16)
                          n324 = Join Numbers(hi=u8 0, lo=w521) -> ((hi.lo)=w519:u16)
                          n325 = Join Numbers(hi=w519, lo=w518) -> ((hi.lo)=w516:u32)
                          n326 = Not Equal?(x=u32 16777215, y=w516) -> (x != y?=w515:bool)
                          n327 = case shown="True" w515 {
                            tunnel: w516 -> [_ w529]
                            frame False {
                            }
                            frame True {
                              n328 = To Double Precision Float(number=w529) -> (double precision float=w528:dbl)
                              n329 = global write "rio_Global.vi" "C_odometer"(w528) -> ()
                            }
                          }
                        }
                      }
                    }
                    frame 1349 {
                      n330 = flat-sequence {
                        tunnel: [w533] -> w530
                        tunnel: [w532] -> w531
                        frame #0 {
                          n331 = local read "FPGA"() -> (w539:refnum<k20>)
                          n332 = xnode "Read/Write Control"("FPGA VI Reference In"=w539) -> ("can 545"=w538:u8[])  [unwired: 1 in, 2 out]
                          n333 = Index Array(array=w538, index #1=0 ("index")) -> (element #1=w545:u8, element #2=w544:u8, element #3=w543:u8, element #4=w542:u8)  [unwired: 3 in]
                          n334 = Join Numbers(hi=w545, lo=w544) -> ((hi.lo)=w541:u16)
                          n335 = Join Numbers(hi=w543, lo=w542) -> ((hi.lo)=w540:u16)
                          n336 = Join Numbers(hi=w541, lo=w540) -> ((hi.lo)=w534:u32)
                          n337 = Array Subset(array=w538, index=4) -> (w532:u8[])  [unwired: 1 in]
                          n338 = feedback #11(u32 0) -> (w535:u32)
                          n339 = feedback-in #11(w534) -> ()
                          n340 = Not Equal?(x=w534, y=w535) -> (x != y?=w533:bool)
                        }
                      }
                      n341 = case shown="True" w530 {
                        tunnel: w531 -> [_ w547]
                        frame False {
                        }
                        frame True {
                          n342 = Index Array(array=w547, index=3) -> (element=w549:u8)
                          n343 = Not Equal?(x=w549, y=u8 255 ("x")) -> (x != y?=w551:bool)
                          n344 = case shown="True" w551 {
                            tunnel: w549 -> [_ w557]
                            frame False {
                            }
                            frame True {
                              n345 = To Double Precision Float(number=w557) -> (double precision float=w556:dbl)
                              n346 = Multiply(x=26.0, y=w556) -> (x*y=w554:dbl)
                              n347 = Divide(x=w554, y=256.0) -> (x/y=w552:dbl)
                              "battery voltage" <- w552
                              n348 = global write "rio_Global.vi" "C_battery voltage"(w552) -> ()
                            }
                          }
                        }
                      }
                    }
                  }
                }
                n349 = Or Array Elements(Boolean array=w226) -> (logical OR=w225:bool)
              }
              frame Disabled {
              }
            }
            "CAN Comm Enabled" <- w224
          }
          frame #2 {
            n350 = global read "rio_Global.vi" "C_VS_CAN"() -> (→"VS_CAN":dbl)
          }
          frame #3 {
            n351 = local read "CAN Comm Enabled"() -> (w559:bool)
            n352 = case shown="True" w559 {
              frame False {
              }
              frame True {
                n353 = Get Date/Time In Seconds() -> (seconds since 1Jan1904=w582:timestamp)
                n354 = global read "rio_Global.vi" "LCM_CAN_T"() -> (w562:T6)
                n355 = To Double Precision Float(number=w582) -> (double precision float=w581:dbl)
                n356 = global read "rio_Global.vi" "C_time"() -> (w577:u32)
                n357 = global read "rio_Global.vi" "C_battery voltage"() -> (w567:dbl)
                n358 = global read "rio_Global.vi" "C_mdps str_ang"() -> (w574:dbl)
                n359 = global read "rio_Global.vi" "C_WHL_SPD_RR"() -> (w566:dbl)
                n360 = global read "rio_Global.vi" "C_WHL_SPD_RL"() -> (w565:dbl)
                n361 = global read "rio_Global.vi" "C_WHL_SPD_FR"() -> (w564:dbl)
                n362 = global read "rio_Global.vi" "C_WHL_SPD_FL"() -> (w563:dbl)
                n363 = global read "rio_Global.vi" "C_mdps torque"() -> (w575:dbl)
                n364 = Unbundle By Name(w562) -> ("hash"=w588:i64)
                n365 = Multiply(x=w581, y=1000000.0) -> (x*y=w579:dbl)
                n366 = global read "rio_Global.vi" "C_odometer"() -> (w569:dbl)
                n367 = global read "rio_Global.vi" "C_yaw_rate"() -> (w576:dbl)
                n368 = global read "rio_Global.vi" "C_lat_accel"() -> (w572:dbl)
                n369 = global read "rio_Global.vi" "C_VS_CAN"() -> (w573:dbl)
                n370 = global read "rio_Global.vi" "C_MCP"() -> (w571:dbl)
                n371 = global read "rio_Global.vi" "C_APV"() -> (w570:dbl)
                n372 = To Quad Integer(1:w579) -> (0:w578:i64)
                n373 = call "hash.vi"("input"=w588) -> ("output"=w587:i64)  [unwired: 10 in]
                n374 = To Double Precision Float(number=w577) -> (double precision float=w586:dbl)
                n375 = global read "rio_Global.vi" "C_tps"() -> (w568:dbl)
                n376 = Bundle By Name(cluster=w562, "hash"=w587, "sys time"=w578, "time"=w586, "yaw_rate"=w576, "mdps torque"=w575, "mdps str_ang"=w574, "VS_CAN"=w573, "lat_accel"=w572, "mcp"=w571, "accel pedal value"=w570, "tps"=w568, "odometer"=w569, "battery voltage"=w567, "WHL_SPD_RR"=w566, "WHL_SPD_RL"=w565, "WHL_SPD_FR"=w564, "WHL_SPD_FL"=w563) -> (w585:T6)
                n377 = Flatten To String(anything=w585, prepend array or string size? (T)=FALSE) -> (data string=w584:string)  [unwired: 2 in, 2 out]
                n378 = global read "rio_Global.vi" "LCM"() -> (w560:T3)
                n379 = call "LCM_send.vi"("DATA"=w584, "ID"="CAN_T", "LCM"=w560) -> ()  [unwired: 6 in, 3 out]
              }
            }
          }
        }
      }
    }
  }
  n380 = flat-sequence {
    frame #0 {
      w593 = FALSE ("GPS init")
      n381 = local write "Manual Steering angle"(0.0 ("steer manual")) -> ()
      n382 = local write "Manual Speed"(0.0 ("Manual Speed")) -> ()
      n383 = local write "Steer input"(TRUE ("Steer input")) -> ()
      n384 = call "car_spec.vi"("Car_name"="Veloster") -> ()  [unwired: 11 in]
      n385 = local write "brake"(w593) -> ()
      n386 = local write "Velocity input"(w593) -> ()
    }
    frame #1 {
      n387 = while {
        stop <- FALSE stop-if-true
        n388 = flat-sequence {
          frame #0 {
            n389 = Wait Until Next ms Multiple(millisecond multiple=u32 10) -> (millisecond timer value=w598:u32)
            n390 = feedback #12(w598) -> (w597:u32)
            n391 = feedback-in #12(w598) -> ()
            n392 = Subtract(x=w598, y=w597) -> (x-y=w596:u32)
            n393 = To Long Integer(number=w596) -> (32bit integer=→"Con_time 10":i32)
          }
          frame #1 {
            n394 = flat-sequence {
              frame #0 {
                n395 = global read "rio_Global.vi" "C_mdps str_ang"() -> (w620:dbl)
                n396 = global read "rio_Global.vi" "C_mdps str_ang"() -> (w619:dbl)
                n397 = global read "rio_Global.vi" "Ref_str_ang"() -> (w618:dbl)
                n398 = Negate(x="Manual Steering angle") -> (-x=w622:dbl)
                n399 = Add(x=w620, y="steer limit") -> (x+y=w626:dbl)
                n400 = Subtract(x=w619, y="steer limit") -> (x-y=w625:dbl)
                n401 = Select(t=w618, s="Steer input", f=w622) -> (s? t:f=w624:dbl)
                n402 = In Range and Coerce(upper limit=w626, x=w624, lower limit=w625) -> (coerced(x)=w617:dbl)  [unwired: 1 out]
                n403 = global write "rio_Global.vi" "steering angle"(w617) -> ()
              }
            }
            n404 = global read "rio_Global.vi" "Ref_VS"() -> (w600:dbl)
            n405 = Select(t=w600, s="Velocity input", f="Manual Speed") -> (s? t:f=w603:dbl)
            n406 = To Long Integer(number=w603) -> (32bit integer=w602:i32)
            n407 = Sign(1:w602) -> (0:w601:i32)
            "P, R, D" <- w601
            n408 = case shown="-1" w601 {
              tunnel: [w608 _ w615] -> w604
              tunnel: w603 -> [w610 _ w614]
              frame -1 {
                n409 = global read "rio_Global.vi" "C_gear selector disp"() -> (w607:u8)
                n410 = Equal?(x=w607, y=u8 7) -> (x = y?=w611:bool)
                n411 = Select(t=w610, s=w611, f=0.0) -> (s? t:f=w608:dbl)
              }
              frame 0, Default {
              }
              frame 1 {
                n412 = global read "rio_Global.vi" "C_gear selector disp"() -> (w613:u8)
                n413 = case shown="0, Default" w613 {
                  tunnel: [_ w616] -> w615
                  tunnel: w614 -> [_ w616]
                  frame 0, Default {
                  }
                  frame 4, 5 {
                  }
                }
              }
            }
            "Ref vel" <- w604
          }
          frame #2 {
            n414 = global read "rio_Global.vi" "Auto"() -> (w636:bool)
            n415 = case shown="True" w636 {
              tunnel: [w639 w674] -> w628
              frame False {
                n416 = global read "rio_Global.vi" "C_VS_CAN"() -> (w638:dbl)
                n417 = global read "rio_Global.vi" "C_gear selector disp"() -> (w637:u8)
                n418 = Absolute Value(x=w638) -> (abs(x)=w642:dbl)
                n419 = Less?(x=w642, y=0.05) -> (x < y?=w640:bool)
                n420 = case shown="True" w640 {
                  tunnel: [_ w646] -> w639
                  tunnel: w637 -> [_ w643]
                  frame False {
                  }
                  frame True {
                    n421 = Sign(1:"Gear Manual") -> (0:w647:i32)
                    n422 = To Long Integer(number=w647) -> (32bit integer=w645:i32)
                    n423 = case shown="1, Default" w645 {
                      tunnel: [w654 w659 w663] -> w646
                      tunnel: w643 -> [w648 w657 w662]
                      frame 0 {
                        n424 = Equal To 0?(x=w648) -> (x = 0?=w652:bool)
                        n425 = Equal?(x=u8 7 ("y"), y=w648) -> (x = y?=w656:bool)
                        n426 = Select(t=-1.0, s=w652, f=1.0) -> (s? t:f=w651:dbl)
                        n427 = Select(t=0.0, s=w656, f=w651) -> (s? t:f=w654:dbl)
                      }
                      frame 1, Default {
                        n428 = Equal To 0?(x=w657) -> (x = 0?=w661:bool)
                        n429 = Select(t=0.0, s=w661, f=1.0 ("t")) -> (s? t:f=w659:dbl)
                      }
                      frame -1 {
                        n430 = case shown="3..5, Default" w662 {
                          tunnel: [-1.0 1.0 0.0] -> w663
                          frame 0, 6, 7 {
                          }
                          frame 1, 2 {
                          }
                          frame 3..5, Default {
                          }
                        }
                      }
                    }
                  }
                }
              }
              frame True {
                n431 = global read "rio_Global.vi" "C_VS_CAN"() -> (w669:dbl)
                n432 = Absolute Value(x=w669) -> (abs(x)=w672:dbl)
                n433 = global read "rio_Global.vi" "C_gear selector disp"() -> (w667:u8)
                n434 = Less?(x=w672, y=0.05) -> (x < y?=w670:bool)
                n435 = global read "rio_Global.vi" "Run"() -> (w668:bool)
                n436 = And(x=w670, y=w668) -> (x .and. y?=w673:bool)
                n437 = case shown="True" w673 {
                  tunnel: [_ w677] -> w674
                  tunnel: w667 -> [_ w675]
                  frame False {
                  }
                  frame True {
                    n438 = local read "P, R, D"() -> (w676:i32)
                    n439 = case shown="-1" w676 {
                      tunnel: [w679 w684 w688] -> w677
                      tunnel: w675 -> [w678 w682 w687]
                      frame -1 {
                        n440 = case shown="0" w678 {
                          tunnel: [-1.0 ("t") 1.0 ("t") _ _] -> w679
                          frame 0 {
                          }
                          frame 1, Default {
                          }
                          frame 4, 8 {
                          }
                          frame 7 {
                          }
                        }
                      }
                      frame 0, Default {
                        n441 = Equal To 0?(x=w682) -> (x = 0?=w686:bool)
                        n442 = Select(t=0.0, s=w686, f=1.0 ("t")) -> (s? t:f=w684:dbl)
                      }
                      frame 1 {
                        n443 = case shown="1, 2" w687 {
                          tunnel: [-1.0 1.0 0.0] -> w688
                          frame 0, 6, 7 {
                          }
                          frame 1, 2 {
                          }
                          frame 3..5, Default {
                          }
                        }
                      }
                    }
                  }
                }
              }
            }
            n444 = Multiply(x=w628, y=250.0 ("S gain")) -> (x*y=w633:dbl)
            n445 = In Range and Coerce(upper limit=500.0, x=w633, lower limit=-500.0) -> (coerced(x)=w630:dbl)  [unwired: 1 out]
            n446 = Add(x=w630, y=1500.0) -> (x+y=w635:dbl)
            n447 = global write "rio_Global.vi" "PWM Shift"(w635) -> ()
          }
          frame #3 {
            n448 = flat-sequence {
              frame #0 {
                n449 = global read "rio_Global.vi" "Auto"() -> (w692:bool)
                n450 = flat-sequence {
                  tunnel: [w703] -> w694
                  frame #0 {
                    n451 = global read "rio_Global.vi" "C_APV"() -> (w708:dbl)
                    n452 = Equal To 0?(x=w708) -> (x = 0?=w710:bool)
                    n453 = case shown="True" w710 {
                      tunnel: [TRUE w718] -> w711
                      frame False {
                        n454 = global write "rio_Global.vi" "T lim counter 2"(u16 300 ("T lim counter 2")) -> ()
                      }
                      frame True {
                        n455 = global read "rio_Global.vi" "T lim counter 2"() -> (w716:u16)
                        n456 = Decrement(x=w716) -> (x-1=w719:u16)
                        n457 = Max & Min(x=u16 0, y=w719) -> (max(x,y)=w717:u16)  [unwired: 1 out]
                        n458 = Not Equal To 0?(x=w717) -> (x != 0?=w718:bool)
                        n459 = global write "rio_Global.vi" "T lim counter 2"(w717) -> ()
                      }
                    }
                    n460 = global read "rio_Global.vi" "Throttle_Enable"() -> (w704:bool)
                    n461 = global read "rio_Global.vi" "C_Brake"() -> (w705:bool)
                    n462 = local read "Ref vel"() -> (w709:dbl)
                    n463 = Not Equal To 0?(x=w709) -> (x != 0?=w713:bool)
                    n464 = Not(x=w705) -> (.not. x?=w712:bool)
                    n465 = global read "rio_Global.vi" "Auto"() -> (w707:bool)
                    n466 = global read "rio_Global.vi" "Run"() -> (w706:bool)
                    n467 = Compound Arithmetic op=AND(w707, w706, w713, w712, w704, w711) -> (w703:bool)
                    n468 = global write "rio_Global.vi" "Solenoid"(w703) -> ()
                  }
                }
                n469 = case shown="True" w692 {
                  tunnel: [w760 w774] -> w693
                  frame False {
                    n470 = global read "rio_Global.vi" "C_MCP"() -> (w757:dbl)
                    n471 = global read "rio_Global.vi" "brake encoder"() -> (w753:dbl)
                    n472 = Multiply(x=w757, y=10.0) -> (x*y=w755:dbl)
                    n473 = Square Root(x=w755) -> (sqrt(x)=w754:dbl)
                    n474 = Not Equal To 0?(x=w753) -> (x != 0?=w759:bool)
                    n475 = Subtract(x=0.0, y=w754) -> (x-y=w761:dbl)
                    n476 = Select(t=w761, s=w759, f=0.0) -> (s? t:f=w760:dbl)
                  }
                  frame True {
                    n477 = global read "rio_Global.vi" "Run"() -> (w763:bool)
                    n478 = case shown="False" w763 {
                      tunnel: [w776 w781] -> w772
                      frame False {
                        n479 = global read "rio_Global.vi" "Const Brk FULL"() -> (w776:dbl)
                      }
                      frame True {
                        n480 = global read "rio_Global.vi" "C_VS_CAN"() -> (w777:dbl)
                        n481 = global read "rio_Global.vi" "Const Brk FULL"() -> (w780:dbl)
                        n482 = local read "Ref vel"() -> (w779:dbl)
                        n483 = Equal To 0?(x=w779) -> (x = 0?=w783:bool)
                        n484 = call "B_control.vi"("Ref vel"=w779, "VS_CAN"=w777) -> ("Ref Brk Enc"=w778:dbl)  [unwired: 17 in]
                        n485 = Select(t=w780, s=w783, f=w778) -> (s? t:f=w782:dbl)
                        n486 = Max & Min(x=w780, y=w782) -> (min(x,y)=w781:dbl)  [unwired: 1 out]
                      }
                    }
                    n487 = global read "rio_Global.vi" "C_MCP"() -> (w768:dbl)
                    n488 = global read "rio_Global.vi" "brake encoder"() -> (w764:dbl)
                    n489 = Multiply(x=w768, y=10.0) -> (x*y=w766:dbl)
                    n490 = Square Root(x=w766) -> (sqrt(x)=w765:dbl)
                    n491 = Subtract(x=w772, y=w765) -> (x-y=w773:dbl)
                    n492 = Equal To 0?(x=w764) -> (x = 0?=w770:bool)
                    n493 = Equal To 0?(x=w772) -> (x = 0?=w771:bool)
                    n494 = And(x=w770, y=w771) -> (x .and. y?=w769:bool)
                    n495 = Select(t=0.0, s=w769, f=w773) -> (s? t:f=w774:dbl)
                  }
                }
                n496 = flat-sequence {
                  tunnel: w693 -> [w748]
                  frame #0 {
                    w723 = 0.2 ("x")
                    n497 = Multiply(x=w748, y=-0.01) -> (x*y=w750:dbl)
                    n498 = In Range and Coerce(upper limit=1.0 ("x"), x=w750, lower limit=-1.0) -> (coerced(x)=w741:dbl)  [unwired: 1 out]
                    n499 = Subtract(x=1.0, y=w723) -> (x-y=w725:dbl)
                    n500 = Multiply(x=w741, y=w723) -> (x*y=w727:dbl)
                    n501 = feedback #13(0.0) -> (w724:dbl)
                    n502 = Multiply(x=w725, y=w724) -> (x*y=w726:dbl)
                    n503 = Add(x=w727, y=w726) -> (x+y=w742:dbl)
                    n504 = feedback-in #13(w742) -> ()
                    n505 = Multiply(x=w741, y=1.8 ("B P gain")) -> (x*y=w722:dbl)
                    n506 = call "deadzone.vi"("min"=-15.0, "max"=15.0, "x"=w742) -> ("dead zone"=w743:dbl)  [unwired: 8 in]
                    n507 = Multiply(x=w743, y=0.1 ("B D gain")) -> (x*y=w721:dbl)
                    n508 = Add(x=w722, y=w721) -> (x+y=w730:dbl)
                    n509 = Multiply(x=w730, y=600.0 ("B gain")) -> (x*y=w738:dbl)
                    n510 = Select(t=w738, s="brake", f="Slide") -> (s? t:f=w736:dbl)
                    n511 = In Range and Coerce(upper limit=500.0, x=w736, lower limit=-500.0) -> (coerced(x)=w735:dbl)  [unwired: 1 out]
                    n512 = Add(x=w735, y=1500.0) -> (x+y=w740:dbl)
                    n513 = global write "rio_Global.vi" "PWM Brake"(w740) -> ()
                  }
                }
                n514 = case shown="True" w694 {
                  tunnel: [w784 w827] -> w702
                  frame False {
                    n515 = flat-sequence {
                      tunnel: [w794] -> w784
                      frame #0 {
                        n516 = global read "rio_Global.vi" "T Lim"() -> (w785:bool)
                        n517 = case shown="True" w785 {
                          selector: w785 -> [_ w790]
                          frame False {
                            n518 = global write "rio_Global.vi" "T lim counter"(u16 0 ("T lim counter")) -> ()
                          }
                          frame True {
                            n519 = global write "rio_Global.vi" "T lim once"(w790) -> ()
                            n520 = global write "rio_Global.vi" "T lim counter 2"(u16 300 ("T lim counter 2")) -> ()
                            n521 = global read "rio_Global.vi" "T lim counter"() -> (w787:u16)
                            n522 = Increment(x=w787) -> (x+1=w792:u16)
                            n523 = Max & Min(x=u16 100, y=w792) -> (min(x,y)=w788:u16)  [unwired: 1 out]
                            n524 = global write "rio_Global.vi" "T lim counter"(w788) -> ()
                          }
                        }
                      }
                      frame #1 {
                        n525 = global read "rio_Global.vi" "T lim once"() -> (w793:bool)
                        n526 = case shown="True" w793 {
                          tunnel: [-1.0 ("t") w799] -> w794
                          frame False {
                          }
                          frame True {
                            n527 = global read "rio_Global.vi" "T lim counter"() -> (w796:u16)
                            n528 = Equal?(x=w796, y=u16 100) -> (x = y?=w798:bool)
                            n529 = Select(t=0.0, s=w798, f=-0.15) -> (s? t:f=w799:dbl)
                          }
                        }
                        n530 = global write "rio_Global.vi" "Throttle_Enable"(w793) -> ()
                      }
                    }
                  }
                  frame True {
                    n531 = global write "rio_Global.vi" "T lim counter"(u16 0 ("T lim counter")) -> ()
                    n532 = global write "rio_Global.vi" "T lim once"(FALSE ("T lim once")) -> ()
                    n533 = global read "rio_Global.vi" "C_VS_CAN"() -> (w807:dbl)
                    n534 = local read "Ref vel"() -> (w806:dbl)
                    n535 = global read "rio_Global.vi" "C_APV"() -> (w803:dbl)
                    n536 = call "T_control.vi"("Ref vel"=w806, "VS_CAN"=w807, "pid gain"=dbl[] [3.0, 0.0, 0.10000000000000003] ("pid gain 1")) -> ("Ref APS"=w804:dbl)  [unwired: 16 in]
                    n537 = global read "rio_Global.vi" "C_APV"() -> (w802:dbl)
                    n538 = Subtract(x=w804, y=w803) -> (x-y=w815:dbl)
                    n539 = flat-sequence {
                      tunnel: w815 -> [w848]
                      tunnel: [w845] -> w822
                      frame #0 {
                        n540 = feedback #14(0.0) -> (w853:dbl)
                        n541 = feedback-in #14(w848) -> ()
                        n542 = Multiply(x=w848, y=0.01) -> (x*y=w849:dbl)
                        n543 = Subtract(x=w848, y=w853) -> (x-y=w852:dbl)
                        n544 = feedback #15(0.0) -> (w844:dbl)
                        n545 = Multiply(x=0.999, y=w844) -> (x*y=w843:dbl)
                        n546 = Divide(x=w852, y=0.01) -> (x/y=w839:dbl)
                        n547 = Add(x=w849, y=w843) -> (x+y=w840:dbl)
                        n548 = feedback-in #15(w840) -> ()
                        n549 = Build Array(w848, w840, w839) -> (w847:dbl[])
                        n550 = Multiply(x=w847, y=dbl[] [8.0, 0.02, 0.4] ("pid gain 2")) -> (x*y=w846:dbl[])
                        n551 = Add Array Elements(numeric array=w846) -> (sum=w845:dbl)
                      }
                    }
                    n552 = Equal To 0?(x=w802) -> (x = 0?=w808:bool)
                    n553 = Greater Than 0?(x=w815) -> (x > 0?=w816:bool)
                    n554 = Less Than 0?(x=w815) -> (x < 0?=w809:bool)
                    n555 = Greater?(x=w802, y=95.0) -> (0:w817:bool)
                    n556 = And(x=w817, y=w816) -> (x .and. y?=w813:bool)
                    n557 = And(x=w808, y=w809) -> (x .and. y?=w814:bool)
                    n558 = Or(x=w813, y=w814) -> (x .or. y?=w812:bool)
                    n559 = Multiply(x=w822, y=0.01) -> (x*y=w820:dbl)
                    n560 = In Range and Coerce(upper limit=1.0 ("x"), x=w820, lower limit=-1.0) -> (coerced(x)=w811:dbl)  [unwired: 1 out]
                    n561 = flat-sequence {
                      tunnel: w811 -> [w829]
                      tunnel: [w835] -> w810
                      frame #0 {
                        w828 = 0.5 ("x")
                        n562 = Multiply(x=w829, y=w828) -> (x*y=w833:dbl)
                        n563 = Subtract(x=1.0, y=w828) -> (x-y=w831:dbl)
                        n564 = feedback #16(0.0) -> (w830:dbl)
                        n565 = Multiply(x=w831, y=w830) -> (x*y=w832:dbl)
                        n566 = Add(x=w833, y=w832) -> (x+y=w835:dbl)
                        n567 = feedback-in #16(w835) -> ()
                      }
                    }
                    n568 = Select(t=0.0 ("f"), s=w812, f=w810) -> (s? t:f=w827:dbl)
                  }
                }
                n569 = Multiply(x=w702, y=500.0 ("T gain")) -> (x*y=w700:dbl)
                n570 = In Range and Coerce(upper limit=500.0, x=w700, lower limit=-500.0) -> (coerced(x)=w696:dbl)  [unwired: 1 out]
                n571 = Add(x=w696, y=1500.0) -> (x+y=w695:dbl)
                n572 = global write "rio_Global.vi" "PWM GAS"(w695) -> ()
              }
              frame #1 {
                w858 = 0.0 ("ref_bkr_enc")
                n573 = Get Date/Time In Seconds() -> (seconds since 1Jan1904=w872:timestamp)
                n574 = global read "rio_Global.vi" "LCM_CON_T"() -> (w857:T7)
                n575 = To Double Precision Float(number=w872) -> (double precision float=w871:dbl)
                n576 = global read "rio_Global.vi" "brake encoder"() -> (w855:dbl)
                n577 = global read "rio_Global.vi" "PWM Brake"() -> (w862:dbl)
                n578 = global read "rio_Global.vi" "PWM GAS"() -> (w860:dbl)
                n579 = global read "rio_Global.vi" "steering angle"() -> (w867:dbl)
                n580 = Unbundle By Name(w857) -> ("hash"=w878:i64)
                n581 = Multiply(x=w871, y=1000000.0) -> (x*y=w869:dbl)
                n582 = global read "rio_Global.vi" "Solenoid"() -> (w866:bool)
                n583 = call "hash.vi"("input"=w878) -> ("output"=w877:i64)  [unwired: 10 in]
                n584 = To Quad Integer(1:w869) -> (0:w868:i64)
                n585 = To Unsigned Byte Integer(number=w855) -> (unsigned 8bit integer=w854:u8)
                n586 = To Unsigned Word Integer(number=w862) -> (unsigned 16bit integer=w861:u16)
                n587 = To Unsigned Word Integer(number=w860) -> (unsigned 16bit integer=w859:u16)
                n588 = local read "Ref vel"() -> (w873:dbl)
                n589 = global read "rio_Global.vi" "T Lim"() -> (w863:bool)
                n590 = global read "rio_Global.vi" "Auto"() -> (w865:bool)
                n591 = global read "rio_Global.vi" "Run"() -> (w864:bool)
                n592 = Bundle(cluster=w857, "hash"=w877, "sys time"=w868, "Auto"=w865, "Run"=w864, "Solenoid"=w866, "T lim"=w863, "brk_enc"=w854, "B PWM"=w861, "T PWM"=w859, "ref_vel"=w873, "ref_bkr_enc"=w858, "ref_apv"=w858, "ref_steer"=w867) -> (w874:T7)
                n593 = Flatten To String(anything=w874, prepend array or string size? (T)=FALSE) -> (data string=w875:string)  [unwired: 2 in, 2 out]
                n594 = global read "rio_Global.vi" "LCM"() -> (w856:T3)
                n595 = call "LCM_send.vi"("DATA"=w875, "ID"="CON_T", "LCM"=w856) -> ()  [unwired: 6 in, 3 out]
              }
            }
          }
        }
      }
    }
  }
  n596 = flat-sequence {
    tunnel: [dbl[] [0.0, 0.0, 0.0, 0.0, 0.0] ("pos(i)")] -> w1
    tunnel: w1 -> [w888]
    frame #0 {
      w884 = 10 ("map")
      w881 = FALSE ("get heading")
      w887 = u64 1
      w886 = 0.0 ("dh_hat")
      n597 = call "getecefdcmref.vi"("map"=w884) -> ("XYZ"=→"ecef ref":dbl[])  [unwired: 10 in, 4 out]
      "vgain" <- 1.0 ("initH")
      "vcount" <- w887
      "hbias" <- w886
      "hcount" <- w887
      "get heading" <- w881
      "get position" <- w881
      "heading error" <- w886
      "h_gps" <- w886
      "rt" <- w886
      "pos error" <- w886
      "map" <- w884
      "POS init" <- TRUE ("pos linit")
    }
    frame #1 {
      n598 = flat-sequence {
        frame #0 {
          n599 = call-poly "VISA Configure Serial Port"("VISA resource name"=refnum<visa-resource-name> "USB0::0x1546::0x01A6::NI-VISA-1::1::RAW", "timeout (10sec)"=u32 1, "baud rate (9600)"=u32 115200) -> ("VISA resource name out"=w964:refnum<visa-resource-name>)  [unwired: 11 in, 1 out]
          n600 = while {
            tunnel: w964 -> [w965]
            stop <- FALSE stop-if-true
            n601 = VISA Read(VISA resource name=w965, byte count=u32 100) -> (read buffer=w966:string)  [unwired: 1 in, 3 out]
            n602 = case shown="Default" w966 {
              selector: w966 -> [_ w970]
              frame "" {
                n603 = Wait (ms)(milliseconds to wait=u32 20) -> ()  [unwired: 1 out]
              }
              frame Default {
                n604 = local read "ecef ref"() -> (w971:dbl[])
                n605 = call "nmea.vi"("ecef ref"=w971, "NMEA"=w970) -> ("output"=w973:dbl[], "type"=w972:u32)  [unwired: 8 in]
                n606 = case shown="1" w972 {
                  tunnel: w973 -> [_ w975 w1008]
                  frame 0, Default {
                  }
                  frame 1 {
                    n607 = global write "rio_Global.vi" "gps_pos 1"(w975) -> ()
                    n608 = Index Array(array=w975, index=1) -> (element=w977:dbl)
                    n609 = Not Equal To 0?(x=w977) -> (x != 0?=w974:bool)
                    n610 = case shown="True" w974 {
                      tunnel: w975 -> [_ w997]
                      frame False {
                      }
                      frame True {
                        n611 = Get Date/Time In Seconds() -> (seconds since 1Jan1904=w982:timestamp)
                        n612 = To Double Precision Float(number=w982) -> (double precision float=w981:dbl)
                        n613 = global read "rio_Global.vi" "LCM_GGA_T"() -> (w1006:T8)
                        n614 = Array To Cluster(array=w997) -> (cluster=w1005:T9)
                        n615 = Unbundle By Name(w1006) -> ("hash"=w1002:i64)
                        n616 = Multiply(x=w981, y=1000000.0) -> (x*y=w979:dbl)
                        n617 = Unbundle(w1005) -> ("output[0]"=w1007:dbl, "output[2]"=w996:dbl, "output[3]"=w995:dbl, "output[4]"=w994:dbl, "output[6]"=w993:dbl, "output[7]"=w991:dbl, "output[8]"=w989:dbl, "output[9]"=w987:dbl, "output[12]"=w986:dbl, "output[13]"=w985:dbl, "output[14]"=w984:dbl)  [unwired: 4 out]
                        n618 = call "hash.vi"("input"=w1002) -> ("output"=w1001:i64)  [unwired: 10 in]
                        n619 = To Quad Integer(1:w979) -> (0:w978:i64)
                        n620 = To Long Integer(number=w993) -> (32bit integer=w992:i32)
                        n621 = To Long Integer(number=w991) -> (32bit integer=w990:i32)
                        n622 = To Long Integer(number=w989) -> (32bit integer=w988:i32)
                        n623 = local read "map"() -> (w983:i32)
                        n624 = Bundle(cluster=w1006, "hash"=w1001, "sys time"=w978, "time"=w1007, "x"=w996, "y"=w995, "h"=w994, "numSV"=w992, "postype"=w990, "lag"=w988, "hordev"=w987, "lat"=w986, "lon"=w985, "hgt"=w984, "map_idx"=w983) -> (w1003:T8)
                        n625 = Flatten To String(anything=w1003, prepend array or string size? (T)=FALSE) -> (data string=w999:string)  [unwired: 2 in, 2 out]
                        n626 = global read "rio_Global.vi" "LCM"() -> (w998:T3)
                        n627 = call "LCM_send.vi"("DATA"=w999, "ID"="GGA_1", "LCM"=w998) -> ()  [unwired: 6 in, 3 out]
                      }
                    }
                  }
                  frame 2 {
                    n628 = flat-sequence {
                      tunnel: w1008 -> [w1010]
                      frame #0 {
                        n629 = Index Array(array=w1010, index=1) -> (element=w1012:dbl)
                        n630 = Not Equal To 0?(x=w1012) -> (x != 0?=w1009:bool)
                        n631 = case shown="True" w1009 {
                          tunnel: w1010 -> [_ w1031]
                          frame False {
                          }
                          frame True {
                            n632 = Get Date/Time In Seconds() -> (seconds since 1Jan1904=w1017:timestamp)
                            n633 = To Double Precision Float(number=w1017) -> (double precision float=w1016:dbl)
                            n634 = global read "rio_Global.vi" "LCM_RMC_T"() -> (w1032:T10)
                            n635 = Unbundle By Name(w1032) -> ("hash"=w1028:i64)
                            n636 = Multiply(x=w1016, y=1000000.0) -> (x*y=w1014:dbl)
                            n637 = Array To Cluster(array=w1031) -> (cluster=w1030:T11)
                            n638 = To Quad Integer(1:w1014) -> (0:w1013:i64)
                            n639 = call "hash.vi"("input"=w1028) -> ("output"=w1027:i64)  [unwired: 10 in]
                            n640 = Unbundle(w1030) -> ("output[0]"=w1022:dbl, "output[2]"=w1021:dbl, "output[4]"=w1020:dbl, "output[5]"=w1019:dbl, "output[6]"=w1018:dbl)  [unwired: 2 out]
                            n641 = Bundle(cluster=w1032, "hash"=w1027, "sys time"=w1013, "time"=w1022, "speed"=w1021, "heading"=w1020, "lat"=w1019, "lon"=w1018) -> (w1023:T10)
                            n642 = Flatten To String(anything=w1023, prepend array or string size? (T)=FALSE) -> (data string=w1025:string)  [unwired: 2 in, 2 out]
                            n643 = global read "rio_Global.vi" "LCM"() -> (w1024:T3)
                            n644 = call "LCM_send.vi"("DATA"=w1025, "ID"="RMC_1", "LCM"=w1024) -> ()  [unwired: 6 in, 3 out]
                          }
                        }
                      }
                    }
                    n645 = global write "rio_Global.vi" "gps_vel 1"(w1008) -> ()
                  }
                }
              }
            }
          }
        }
      }
      n646 = flat-sequence {
        frame #0 {
          n647 = call-poly "VISA Configure Serial Port"("VISA resource name"=refnum<visa-resource-name> "USB0::0x1546::0x01A6::NI-VISA-0::1::RAW", "timeout (10sec)"=u32 1, "baud rate (9600)"=u32 115200) -> ("VISA resource name out"=w892:refnum<visa-resource-name>)  [unwired: 11 in, 1 out]
          n648 = while {
            tunnel: w892 -> [w893]
            stop <- FALSE stop-if-true
            n649 = VISA Read(VISA resource name=w893, byte count=u32 100) -> (read buffer=w894:string)  [unwired: 1 in, 3 out]
            n650 = case shown="Default" w894 {
              selector: w894 -> [_ w898]
              frame "" {
                n651 = Wait (ms)(milliseconds to wait=u32 20) -> ()  [unwired: 1 out]
              }
              frame Default {
                n652 = local read "ecef ref"() -> (w899:dbl[])
                n653 = call "nmea.vi"("ecef ref"=w899, "NMEA"=w898) -> ("output"=w901:dbl[], "type"=w900:u32)  [unwired: 8 in]
                n654 = case shown="1" w900 {
                  tunnel: w901 -> [_ w903 w936]
                  frame 0, Default {
                  }
                  frame 1 {
                    n655 = global write "rio_Global.vi" "gps_pos 2"(w903) -> ()
                    n656 = Index Array(array=w903, index=1) -> (element=w905:dbl)
                    n657 = Not Equal To 0?(x=w905) -> (x != 0?=w902:bool)
                    n658 = case shown="True" w902 {
                      tunnel: w903 -> [_ w925]
                      frame False {
                      }
                      frame True {
                        n659 = Get Date/Time In Seconds() -> (seconds since 1Jan1904=w910:timestamp)
                        n660 = To Double Precision Float(number=w910) -> (double precision float=w909:dbl)
                        n661 = global read "rio_Global.vi" "LCM_GGA_T"() -> (w934:T8)
                        n662 = Array To Cluster(array=w925) -> (cluster=w933:T9)
                        n663 = Unbundle By Name(w934) -> ("hash"=w930:i64)
                        n664 = Multiply(x=w909, y=1000000.0) -> (x*y=w907:dbl)
                        n665 = Unbundle(w933) -> ("output[0]"=w935:dbl, "output[2]"=w924:dbl, "output[3]"=w923:dbl, "output[4]"=w922:dbl, "output[6]"=w921:dbl, "output[7]"=w919:dbl, "output[8]"=w917:dbl, "output[9]"=w915:dbl, "output[12]"=w914:dbl, "output[13]"=w913:dbl, "output[14]"=w912:dbl)  [unwired: 4 out]
                        n666 = call "hash.vi"("input"=w930) -> ("output"=w929:i64)  [unwired: 10 in]
                        n667 = To Quad Integer(1:w907) -> (0:w906:i64)
                        n668 = To Long Integer(number=w921) -> (32bit integer=w920:i32)
                        n669 = To Long Integer(number=w919) -> (32bit integer=w918:i32)
                        n670 = To Long Integer(number=w917) -> (32bit integer=w916:i32)
                        n671 = local read "map"() -> (w911:i32)
                        n672 = Bundle(cluster=w934, "hash"=w929, "sys time"=w906, "time"=w935, "x"=w924, "y"=w923, "h"=w922, "numSV"=w920, "postype"=w918, "lag"=w916, "hordev"=w915, "lat"=w914, "lon"=w913, "hgt"=w912, "map_idx"=w911) -> (w931:T8)
                        n673 = Flatten To String(anything=w931, prepend array or string size? (T)=FALSE) -> (data string=w927:string)  [unwired: 2 in, 2 out]
                        n674 = global read "rio_Global.vi" "LCM"() -> (w926:T3)
                        n675 = call "LCM_send.vi"("DATA"=w927, "ID"="GGA_2", "LCM"=w926) -> ()  [unwired: 6 in, 3 out]
                      }
                    }
                  }
                  frame 2 {
                    n676 = flat-sequence {
                      tunnel: w936 -> [w938]
                      frame #0 {
                        n677 = Index Array(array=w938, index=1) -> (element=w940:dbl)
                        n678 = Not Equal To 0?(x=w940) -> (x != 0?=w937:bool)
                        n679 = case shown="True" w937 {
                          tunnel: w938 -> [_ w959]
                          frame False {
                          }
                          frame True {
                            n680 = Get Date/Time In Seconds() -> (seconds since 1Jan1904=w945:timestamp)
                            n681 = To Double Precision Float(number=w945) -> (double precision float=w944:dbl)
                            n682 = global read "rio_Global.vi" "LCM_RMC_T"() -> (w960:T10)
                            n683 = Unbundle By Name(w960) -> ("hash"=w956:i64)
                            n684 = Multiply(x=w944, y=1000000.0) -> (x*y=w942:dbl)
                            n685 = Array To Cluster(array=w959) -> (cluster=w958:T11)
                            n686 = To Quad Integer(1:w942) -> (0:w941:i64)
                            n687 = call "hash.vi"("input"=w956) -> ("output"=w955:i64)  [unwired: 10 in]
                            n688 = Unbundle(w958) -> ("output[0]"=w950:dbl, "output[2]"=w949:dbl, "output[4]"=w948:dbl, "output[5]"=w947:dbl, "output[6]"=w946:dbl)  [unwired: 2 out]
                            n689 = Bundle(cluster=w960, "hash"=w955, "sys time"=w941, "time"=w950, "speed"=w949, "heading"=w948, "lat"=w947, "lon"=w946) -> (w951:T10)
                            n690 = Flatten To String(anything=w951, prepend array or string size? (T)=FALSE) -> (data string=w953:string)  [unwired: 2 in, 2 out]
                            n691 = global read "rio_Global.vi" "LCM"() -> (w952:T3)
                            n692 = call "LCM_send.vi"("DATA"=w953, "ID"="RMC_2", "LCM"=w952) -> ()  [unwired: 6 in, 3 out]
                          }
                        }
                      }
                    }
                    n693 = global write "rio_Global.vi" "gps_vel 2"(w936) -> ()
                  }
                }
              }
            }
          }
        }
      }
      n694 = while {
        shift-right: [w1033] -> _
        shift-left: w888 -> [w1034]
        stop <- FALSE stop-if-true
        n695 = flat-sequence {
          tunnel: [w1045] -> w1037
          tunnel: w1034 -> [w1045]
          tunnel: w1037 -> [w1048]
          tunnel: [w1047] -> w1036
          tunnel: [w1047] -> w1035
          tunnel: [w1461] -> w1033
          tunnel: w1036 -> [w1462]
          tunnel: w1035 -> [w1461]
          frame #0 {
            n696 = global read "rio_Global.vi" "C_ts"() -> (→"dt":dbl)
            n697 = Wait Until Next ms Multiple(millisecond multiple=u32 10) -> (millisecond timer value=w1043:u32)
            n698 = feedback #17(w1043) -> (w1042:u32)
            n699 = feedback-in #17(w1043) -> ()
            n700 = Subtract(x=w1043, y=w1042) -> (x-y=w1041:u32)
            n701 = To Long Integer(number=w1041) -> (32bit integer=→"Pos_time 10":i32)
          }
          frame #1 {
            n702 = flat-sequence {
              tunnel: w1048 -> [w1055]
              tunnel: [w1055] -> w1046
              tunnel: [w1178] -> w1047
              tunnel: w1046 -> [w1179]
              frame #0 {
                n703 = disable-structure shown="Enabled" {
                  disable-tunnel: [w1075 w1076] -> w1050
                  disable-tunnel: [w1056 w1077] -> w1049
                  frame Enabled {
                    n704 = global read "rio_Global.vi" "gps_pos 1"() -> (w1072:dbl[])
                    n705 = global read "rio_Global.vi" "gps_pos 2"() -> (w1059:dbl[])
                    n706 = Add(x=w1072, y=w1059) -> (x+y=w1074:dbl[])
                    n707 = Index Array(array=w1072, index #1=0 ("index")) -> (element #1=w1071:dbl, element #2=w1070:dbl)  [unwired: 1 in]
                    n708 = Index Array(array=w1059, index #1=0 ("index")) -> (element #1=w1060:dbl, element #2=w1061:dbl)  [unwired: 1 in]
                    n709 = feedback #18(w1071) -> (w1069:dbl)
                    n710 = feedback-in #18(w1071) -> ()
                    n711 = feedback #19(w1060) -> (w1062:dbl)
                    n712 = feedback-in #19(w1060) -> ()
                    n713 = Not Equal?(x=w1071, y=w1069) -> (x != y?=w1068:bool)
                    n714 = Not Equal?(x=w1060, y=w1062) -> (x != y?=w1063:bool)
                    n715 = Not Equal To 0?(x=w1070) -> (x != 0?=w1067:bool)
                    n716 = Not Equal To 0?(x=w1061) -> (x != 0?=w1064:bool)
                    n717 = And(x=w1068, y=w1067) -> (x .and. y?=w1057:bool)
                    n718 = And(x=w1063, y=w1064) -> (x .and. y?=w1058:bool)
                    n719 = And(x=w1057, y=w1058) -> (x .and. y?=w1075:bool)
                    n720 = Multiply(x=w1074, y=0.5) -> (x*y=w1056:dbl[])
                  }
                  frame Disabled {
                    n721 = global read "rio_Global.vi" "gps_pos 1"() -> (w1077:dbl[])
                    n722 = Index Array(array=w1077, index #1=0 ("index")) -> (element #1=w1083:dbl, element #2=w1082:dbl)  [unwired: 1 in]
                    n723 = feedback #20(w1083) -> (w1081:dbl)
                    n724 = feedback-in #20(w1083) -> ()
                    n725 = Not Equal?(x=w1083, y=w1081) -> (x != y?=w1080:bool)
                    n726 = Not Equal To 0?(x=w1082) -> (x != 0?=w1079:bool)
                    n727 = And(x=w1080, y=w1079) -> (x .and. y?=w1076:bool)
                  }
                }
                "pos_gps" <- w1049
                n728 = disable-structure shown="Enabled" {
                  disable-tunnel: [w1129 w1160] -> w1054
                  disable-tunnel: [w1128 w1139] -> w1053
                  disable-tunnel: [w1100 w1150] -> w1052
                  disable-tunnel: [w1088 w1145] -> w1051
                  frame Enabled {
                    n729 = global read "rio_Global.vi" "gps_vel 1"() -> (w1127:dbl[])
                    n730 = global read "rio_Global.vi" "gps_vel 2"() -> (w1106:dbl[])
                    n731 = Index Array(array=w1127, index #1=0 ("index"), index #2=1 ("index"), index #3=4 ("index"), index #4=2 ("index")) -> (element #1=w1118:dbl, element #2=w1123:dbl, element #3=w1120:dbl, element #4=w1092:dbl)
                    n732 = Index Array(array=w1106, index #1=0 ("index"), index #2=1 ("index"), index #3=4 ("index"), index #4=2 ("index")) -> (element #1=w1115:dbl, element #2=w1110:dbl, element #3=w1113:dbl, element #4=w1091:dbl)
                    n733 = global read "rio_Global.vi" "C_VS_CAN"() -> (w1085:dbl)
                    n734 = global read "rio_Global.vi" "C_VS_CAN"() -> (w1132:dbl)
                    n735 = Add(x=w1092, y=w1091) -> (x+y=w1090:dbl)
                    n736 = call "angleconv.vi"("deg"=w1120) -> ("rad"=w1103:dbl)  [unwired: 9 in, 1 out]
                    n737 = call "angleconv.vi"("deg"=w1113) -> ("rad"=w1102:dbl)  [unwired: 9 in, 1 out]
                    n738 = Not Equal To 0?(x=w1110) -> (x != 0?=w1111:bool)
                    n739 = feedback #21(0.0 ("Real Matrix Element")) -> (w1117:dbl)
                    n740 = feedback-in #21(w1118) -> ()
                    n741 = feedback #22(0.0 ("Real Matrix Element")) -> (w1116:dbl)
                    n742 = feedback-in #22(w1115) -> ()
                    n743 = Not Equal?(x=w1118, y=w1117) -> (x != y?=w1124:bool)
                    n744 = Not Equal?(x=w1115, y=w1116) -> (x != y?=w1109:bool)
                    n745 = Greater Or Equal To 0?(x=w1132) -> (x >= 0?=w1133:bool)
                    n746 = Not Equal To 0?(x=w1123) -> (x != 0?=w1122:bool)
                    n747 = Absolute Value(x=w1085) -> (abs(x)=w1084:dbl)
                    n748 = Multiply(x=w1090, y=0.5) -> (x*y=w1099:dbl)
                    n749 = call "headingweightsum.vi"("a"=0.5, "h1"=w1102, "h2"=w1103) -> ("a*h2+(1-a)*h1"=w1131:dbl)  [unwired: 8 in]
                    n750 = And(x=w1124, y=w1122) -> (x .and. y?=w1105:bool)
                    n751 = And(x=w1109, y=w1111) -> (x .and. y?=w1104:bool)
                    n752 = Divide(x=w1099, y=w1084) -> (x/y=w1100:dbl)
                    n753 = Select(t=0.0, s=w1133, f=3.141592653589793) -> (s? t:f=w1130:dbl)
                    n754 = Decrement(x=w1100) -> (x-1=w1096:dbl)
                    n755 = call "headingoperater.vi"("h1"=w1130, "h2"=w1131) -> ("h2-h1"=w1129:dbl)  [unwired: 8 in, 1 out]
                    n756 = And(x=w1105, y=w1104) -> (x .and. y?=w1128:bool)
                    n757 = Absolute Value(x=w1096) -> (abs(x)=w1097:dbl)
                    n758 = Greater?(x=w1084, y=15.0) -> (0:w1086:bool)
                    n759 = Less?(x=w1097, y=0.05) -> (x < y?=w1089:bool)
                    n760 = Compound Arithmetic op=AND(w1086, w1089, w1128) -> (w1088:bool)
                  }
                  frame Disabled {
                    n761 = global read "rio_Global.vi" "gps_vel 1"() -> (w1159:dbl[])
                    n762 = global read "rio_Global.vi" "C_VS_CAN"() -> (w1143:dbl)
                    n763 = global read "rio_Global.vi" "C_VS_CAN"() -> (w1162:dbl)
                    n764 = Index Array(array=w1159, index #1=0 ("index"), index #2=1 ("index"), index #3=4 ("index"), index #4=2 ("index")) -> (element #1=w1138:dbl, element #2=w1155:dbl, element #3=w1152:dbl, element #4=w1141:dbl)
                    n765 = Greater Or Equal To 0?(x=w1162) -> (x >= 0?=w1163:bool)
                    n766 = Absolute Value(x=w1143) -> (abs(x)=w1142:dbl)
                    n767 = feedback #23(w1138) -> (w1151:dbl)
                    n768 = feedback-in #23(w1138) -> ()
                    n769 = Divide(x=w1141, y=w1142) -> (x/y=w1150:dbl)
                    n770 = call "angleconv.vi"("deg"=w1152) -> ("rad"=w1140:dbl)  [unwired: 9 in, 1 out]
                    n771 = Select(t=0.0, s=w1163, f=3.141592653589793) -> (s? t:f=w1161:dbl)
                    n772 = Not Equal?(x=w1138, y=w1151) -> (x != y?=w1156:bool)
                    n773 = Decrement(x=w1150) -> (x-1=w1147:dbl)
                    n774 = Not Equal To 0?(x=w1155) -> (x != 0?=w1154:bool)
                    n775 = call "headingoperater.vi"("h1"=w1161, "h2"=w1140) -> ("h2-h1"=w1160:dbl)  [unwired: 8 in, 1 out]
                    n776 = And(x=w1156, y=w1154) -> (x .and. y?=w1139:bool)
                    n777 = Absolute Value(x=w1147) -> (abs(x)=w1148:dbl)
                    n778 = Greater?(x=w1142, y=15.0) -> (0:w1136:bool)
                    n779 = Less?(x=w1148, y=0.05) -> (x < y?=w1137:bool)
                    n780 = Compound Arithmetic op=AND(w1139, w1137, w1136) -> (w1145:bool)
                  }
                }
                n781 = local write "get position"(w1050) -> ()
                n782 = local write "h_gps"(w1054) -> ()
                n783 = case shown="True" w1051 {
                  tunnel: w1052 -> [_ w1173]
                  frame False {
                  }
                  frame True {
                    w1167 = u64 18446744073709551615
                    n784 = local read "vcount"() -> (w1170:u64)
                    n785 = local read "vgain"() -> (w1175:dbl)
                    n786 = Increment(x=w1170) -> (x+1=w1169:u64)
                    n787 = Multiply(x=w1175, y=w1170) -> (x*y=w1174:dbl)
                    n788 = Not Equal?(x=w1170, y=w1167) -> (x != y?=w1168:bool)
                    n789 = Add(x=w1173, y=w1174) -> (x+y=w1172:dbl)
                    n790 = Select(t=w1169, s=w1168, f=w1167) -> (s? t:f=w1166:u64)
                    n791 = Divide(x=w1172, y=w1166) -> (x/y=w1171:dbl)
                    n792 = local write "vcount"(w1166) -> ()
                    n793 = local write "vgain"(w1171) -> ()
                  }
                }
                n794 = local write "get heading"(w1053) -> ()
              }
              frame #1 {
                n795 = local read "dt"() -> (w1177:dbl)
                n796 = Greater Than 0?(x=w1177) -> (x > 0?=w1176:bool)
                n797 = case shown="True" w1176 {
                  tunnel: w1179 -> [w1180 w1183]
                  tunnel: [w1180 w1182] -> w1178
                  frame False {
                  }
                  frame True {
                    n798 = flat-sequence {
                      tunnel: w1183 -> [w1217]
                      tunnel: [w1195] -> w1181
                      tunnel: [w1245] -> w1182
                      tunnel: w1181 -> [w1244]
                      frame #0 {
                        n799 = global read "rio_Global.vi" "C_VS_CAN"() -> (w1185:dbl)
                        n800 = Equal To 0?(x=w1185) -> (x = 0?=w1187:bool)
                        n801 = case shown="False" w1187 {
                          tunnel: [w1219 _] -> w1186
                          frame False {
                            n802 = global read "rio_Global.vi" "C_yaw_rate"() -> (w1218:dbl)
                            n803 = local read "hbias"() -> (w1222:dbl)
                            n804 = Subtract(x=w1218, y=w1222) -> (x-y=w1220:dbl)
                            n805 = Negate(x=w1220) -> (-x=w1221:dbl)
                            n806 = call "angleconv.vi"("deg"=w1221) -> ("rad"=w1219:dbl)  [unwired: 9 in, 1 out]
                          }
                          frame True {
                            w1226 = u64 18446744073709551615
                            n807 = local read "hcount"() -> (w1229:u64)
                            n808 = local read "hbias"() -> (w1232:dbl)
                            n809 = Increment(x=w1229) -> (x+1=w1228:u64)
                            n810 = global read "rio_Global.vi" "C_yaw_rate"() -> (w1223:dbl)
                            n811 = Not Equal?(x=w1229, y=w1226) -> (x != y?=w1227:bool)
                            n812 = Multiply(x=w1232, y=w1229) -> (x*y=w1231:dbl)
                            n813 = Add(x=w1223, y=w1231) -> (x+y=w1230:dbl)
                            n814 = Select(t=w1228, s=w1227, f=w1226) -> (s? t:f=w1225:u64)
                            n815 = local write "hcount"(w1225) -> ()
                            n816 = Divide(x=w1230, y=w1225) -> (x/y=w1224:dbl)
                            n817 = local write "hbias"(w1224) -> ()
                          }
                        }
                        n818 = global read "rio_Global.vi" "C_VS_CAN"() -> (w1184:dbl)
                        n819 = local read "vgain"() -> (w1190:dbl)
                        n820 = Multiply(x=w1184, y=w1190) -> (x*y=w1189:dbl)
                        n821 = Divide(x=w1189, y=3.6) -> (x/y=w1188:dbl)
                        n822 = Index Array(array=w1217, index #1=0 ("index"), index #2=3 ("index"), index #3=1 ("index"), index #4=3 ("index")) -> (element #1=w1211:dbl, element #2=w1209:dbl, element #3=w1205:dbl, element #4=w1200:dbl)
                        n823 = local read "dt"() -> (w1214:dbl)
                        n824 = local read "dt"() -> (w1198:dbl)
                        n825 = Multiply(x=w1188, y=w1214) -> (x*y=w1210:dbl)
                        n826 = Multiply(x=w1198, y=w1186) -> (x*y=w1191:dbl)
                        n827 = Cosine(x=w1209) -> (cos(x)=w1215:dbl)
                        n828 = Sine(x=w1209) -> (sin(x)=w1208:dbl)
                        n829 = Multiply(x=w1215, y=w1210) -> (x*y=w1212:dbl)
                        n830 = Multiply(x=w1210, y=w1208) -> (x*y=w1207:dbl)
                        n831 = local write "rt"(w1191) -> ()
                        n832 = Add(x=w1211, y=w1212) -> (x+y=w1204:dbl)
                        n833 = Add(x=w1207, y=w1205) -> (x+y=w1203:dbl)
                        n834 = call "headingoperater.vi"("h1"=w1191, "h2"=w1200) -> ("h2+h1"=w1199:dbl)  [unwired: 8 in, 1 out]
                        n835 = Build Array(w1204, w1203, w1188, w1199, w1186) -> (w1195:dbl[])
                        n836 = Index Array(array=w1195, index=3) -> (element=w1194:dbl)
                        n837 = local read "h_gps"() -> (w1193:dbl)
                        n838 = call "headingoperater.vi"("h1"=w1194, "h2"=w1193) -> ("h2-h1"=w1197:dbl)  [unwired: 8 in, 1 out]
                        n839 = Absolute Value(x=w1197) -> (abs(x)=w1192:dbl)
                        n840 = local write "heading error"(w1192) -> ()
                      }
                      frame #1 {
                        n841 = local read "get heading"() -> (w1252:bool)
                        n842 = local read "get position"() -> (w1251:bool)
                        n843 = local read "POS init"() -> (w1237:bool)
                        n844 = case shown="False" w1237 {
                          tunnel: w1252 -> [w1255 w1262]
                          tunnel: w1251 -> [w1259 w1261]
                          tunnel: [w1253 w1260] -> w1247
                          frame False {
                            n845 = local read "heading error"() -> (w1256:dbl)
                            n846 = Less?(x=w1256, y=0.05) -> (x < y?=w1257:bool)
                            n847 = And(x=w1255, y=w1257) -> (x .and. y?=w1254:bool)
                            n848 = Or(x=w1254, y=w1259) -> (x .or. y?=w1253:bool)
                          }
                          frame True {
                            n849 = disable-structure shown="Enabled" {
                              disable-tunnel: w1262 -> [w1265 w1267]
                              disable-tunnel: w1261 -> [w1264 w1266]
                              disable-tunnel: [w1263 w1268] -> w1260
                              frame Disabled {
                                n850 = And(x=w1265, y=w1264) -> (x .and. y?=w1263:bool)
                              }
                              frame Enabled {
                                n851 = Or(x=w1267, y=w1266) -> (x .or. y?=w1268:bool)
                              }
                            }
                          }
                        }
                        n852 = global read "rio_Global.vi" "C_VS_CAN"() -> (w1250:dbl)
                        n853 = local read "heading error"() -> (w1240:dbl)
                        n854 = Absolute Value(x=w1250) -> (abs(x)=w1249:dbl)
                        n855 = local read "POS init"() -> (w1238:bool)
                        n856 = Greater?(x=w1249, y=5.0) -> (0:w1246:bool)
                        n857 = Less?(x=w1240, y=1.0) -> (x < y?=w1239:bool)
                        n858 = Or(x=w1239, y=w1238) -> (x .or. y?=w1241:bool)
                        n859 = And(x=w1247, y=w1246) -> (x .and. y?=w1242:bool)
                        n860 = And(x=w1242, y=w1241) -> (x .and. y?=w1235:bool)
                        n861 = Select(t=FALSE, s="GPS init", f=w1235) -> (s? t:f=w1234:bool)
                        n862 = case shown="True" w1234 {
                          tunnel: [w1272 w1301] -> w1245
                          tunnel: w1244 -> [w1273 w1304]
                          frame False {
                            n863 = global read "rio_Global.vi" "C_VS_CAN"() -> (w1276:dbl)
                            n864 = local read "POS init"() -> (w1275:bool)
                            n865 = Equal To 0?(x=w1276) -> (x = 0?=w1274:bool)
                            n866 = local read "GPS init"() -> (w1269:bool)
                            n867 = And(x=w1275, y=w1274) -> (x .and. y?=w1271:bool)
                            n868 = Or(x=w1271, y=w1269) -> (x .or. y?=w1270:bool)
                            n869 = case shown="True" w1270 {
                              tunnel: w1273 -> [w1277 w1278]
                              tunnel: [w1277 w1280] -> w1272
                              tunnel: w1269 -> [_ w1279]
                              frame False {
                              }
                              frame True {
                                n870 = case shown="True" w1279 {
                                tunnel: [w1291 w1300] -> w1280
                                tunnel: w1278 -> [w1286 w1294]
                                frame True {
                                n871 = Index Array(array=w1286, index #1=2 ("index")) -> (element #2=w1281:dbl, element #3=w1284:dbl)  [unwired: 2 in, 1 out]
                                n872 = local read "pos_gps"() -> (w1287:dbl[])
                                n873 = local write "GPS init"(FALSE ("GPS init")) -> ()
                                n874 = Index Array(array=w1287, index #1=2 ("index")) -> (element #1=w1289:dbl, element #2=w1288:dbl)  [unwired: 1 in]
                                n875 = local read "h_gps"() -> (w1282:dbl)
                                n876 = Build Array(w1289, w1288, w1281, w1282, w1284) -> (w1291:dbl[])
                                }
                                frame False {
                                w1293 = 0.0 ("element")
                                n877 = Index Array(array=w1294, index=3) -> (element=w1292:dbl)
                                n878 = local read "pos_gps"() -> (w1296:dbl[])
                                n879 = Index Array(array=w1296, index #1=2 ("index")) -> (element #1=w1298:dbl, element #2=w1297:dbl)  [unwired: 1 in]
                                n880 = Build Array(w1298, w1297, w1293, w1292, w1293) -> (w1300:dbl[])
                                }
                                }
                              }
                            }
                          }
                          frame True {
                            n881 = flat-sequence {
                              tunnel: w1304 -> [w1305]
                              tunnel: [w1305] -> w1303
                              tunnel: w1303 -> [w1346]
                              tunnel: [w1346] -> w1302
                              tunnel: w1302 -> [w1373]
                              tunnel: [w1377] -> w1301
                              frame #0 {
                                w1314 = 0.0 ("element")
                                w1318 = 0.0 ("element")
                                w1320 = 0.0 ("element")
                                w1322 = 0.0 ("element")
                                w1324 = 0.0 ("element")
                                n882 = Index Array(array=w1305, index #1=3 ("index"), index #2=2 ("index"), index #3=3 ("index"), index #4=2 ("index")) -> (element #1=w1334:dbl, element #2=w1336:dbl, element #3=w1339:dbl, element #4=w1328:dbl)
                                n883 = Negate(x=w1336) -> (-x=w1335:dbl)
                                n884 = Sine & Cosine(0:w1339) -> (1:w1331:dbl, 2:w1329:dbl)
                                n885 = Multiply(x=w1335, y=w1331) -> (x*y=w1332:dbl)
                                n886 = Multiply(x=w1329, y=w1328) -> (x*y=w1327:dbl)
                                n887 = Cosine(x=w1334) -> (cos(x)=w1333:dbl)
                                n888 = Build Array(w1324, w1324, w1333, w1332, 0.0 ("element")) -> (w1326:dbl[])
                                n889 = Build Array(w1322, w1322, w1331, w1327, 0.0 ("element")) -> (w1325:dbl[])
                                n890 = Build Array(w1320, w1320, w1320, w1320, w1320) -> (w1319:dbl[])
                                n891 = Build Array(w1318, w1318, w1318, w1318, 1.0 ("element")) -> (w1316:dbl[])
                                n892 = Build Array(w1314, w1314, w1314, w1314, w1314) -> (w1315:dbl[])
                                n893 = Build Array(w1326, w1325, w1319, w1316, w1315) -> (w1312:dbl[][])
                                n894 = call-poly <vilib>:"Array To Matrix.vi"("Real 2D Array"=w1312) -> ("Real Matrix"=w1310:T12)
                                n895 = global read "rio_Global.vi" "P"() -> (w1313:T12)
                                n896 = Transpose Matrix(1:w1310) -> (0:w1309:T12)
                                n897 = call-poly <vilib>:"Multiply.vi"("Real Matrix B"=w1313, "Real Matrix A"=w1310) -> ("A * B"=w1311:T12)
                                n898 = call-poly <vilib>:"Multiply.vi"("Real Matrix B"=w1309, "Real Matrix A"=w1311) -> ("A * B"=w1308:T12)
                                n899 = global read "rio_Global.vi" "Q"() -> (w1307:T12)
                                n900 = call-poly <vilib>:"Add.vi"("Real Matrix B"=w1307, "Real Matrix A"=w1308) -> ("A + B"=w1306:T12)
                                n901 = global write "rio_Global.vi" "Pp"(w1306) -> ()
                              }
                              frame #1 {
                                n902 = global read "rio_Global.vi" "Pp"() -> (w1371:T12)
                                n903 = global read "rio_Global.vi" "H"() -> (w1370:T12)
                                n904 = Array Subset(array=w1346, index=0, length=2) -> (w1353:dbl[])
                                n905 = local read "pos_gps"() -> (w1349:dbl[])
                                n906 = call-poly <vilib>:"Multiply.vi"("Real Matrix B"=w1371, "Real Matrix A"=w1370) -> ("A * B"=w1369:T12)
                                n907 = Transpose Matrix(1:w1370) -> (0:w1368:T12)
                                n908 = call-poly <vilib>:"Multiply.vi"("Real Matrix B"=w1368, "Real Matrix A"=w1369) -> ("A * B"=w1367:T12)
                                n909 = Array Subset(array=w1349, index=2, length=2) -> (w1352:dbl[])
                                n910 = Subtract(x=w1352, y=w1353) -> (x-y=w1354:dbl[])
                                n911 = global read "rio_Global.vi" "H"() -> (w1365:T12)
                                n912 = global read "rio_Global.vi" "R"() -> (w1366:T12)
                                n913 = global read "rio_Global.vi" "Pp"() -> (w1364:T12)
                                n914 = call-poly <vilib>:"Add.vi"("Real Matrix B"=w1366, "Real Matrix A"=w1367) -> ("A + B"=w1361:T12)
                                n915 = Square(x=w1354) -> (x^2=w1355:dbl[])
                                n916 = Transpose Matrix(1:w1365) -> (0:w1363:T12)
                                n917 = local read "heading error"() -> (w1358:dbl)
                                n918 = call-poly <vilib>:"Multiply.vi"("Real Matrix B"=w1363, "Real Matrix A"=w1364) -> ("A * B"=w1362:T12)
                                n919 = Add Array Elements(numeric array=w1355) -> (sum=w1356:dbl)
                                n920 = call-poly <vilib>:"Inverse Matrix.vi"("Input Matrix"=w1361) -> ("Inverse Matrix"=w1360:T12)  [unwired: 1 in, 1 out]
                                n921 = call-poly <vilib>:"Multiply.vi"("Real Matrix B"=w1360, "Real Matrix A"=w1362) -> ("A * B"=w1359:T12)
                                n922 = Square Root(x=w1356) -> (sqrt(x)=w1345:dbl)
                                n923 = global write "rio_Global.vi" "K"(w1359) -> ()
                                n924 = Less?(x=w1345, y=2.5) -> (x < y?=w1342:bool)
                                n925 = Less?(x=w1358, y=0.05) -> (x < y?=w1343:bool)
                                n926 = And(x=w1343, y=w1342) -> (x .and. y?=w1341:bool)
                                n927 = case shown="True" w1341 {
                                frame False {
                                }
                                frame True {
                                n928 = local write "POS init"(FALSE ("Kalman init")) -> ()
                                }
                                }
                              }
                              frame #2 {
                                n929 = disable-structure shown="Enabled" {
                                disable-tunnel: [w1395 w1397] -> w1375
                                disable-tunnel: w1373 -> [_ w1406]
                                frame Disabled {
                                n930 = local read item#-1() -> (w1395)
                                }
                                frame Enabled {
                                n931 = Array Subset(array=w1406, index=0, length=2) -> (w1404:dbl[])
                                n932 = local read "pos_gps"() -> (w1409:dbl[])
                                n933 = Array Subset(array=w1409, index=2, length=2) -> (w1405:dbl[])
                                n934 = Subtract(x=w1405, y=w1404) -> (x-y=w1403:dbl[])
                                n935 = Square(x=w1403) -> (x^2=w1402:dbl[])
                                n936 = Add Array Elements(numeric array=w1402) -> (sum=w1401:dbl)
                                n937 = disable-structure shown="Enabled" {
                                disable-tunnel: [w1412 TRUE ("Kalman init")] -> w1399
                                frame Disabled {
                                n938 = local read item#-1() -> (w1412)
                                }
                                frame Enabled {
                                }
                                }
                                n939 = Square Root(x=w1401) -> (sqrt(x)=w1396:dbl)
                                n940 = local write "pos error"(w1396) -> ()
                                n941 = Less?(x=w1396, y=3.0) -> (x < y?=w1398:bool)
                                n942 = Or(x=w1399, y=w1398) -> (x .or. y?=w1397:bool)
                                }
                                }
                                n943 = disable-structure shown="Enabled" {
                                disable-tunnel: [w1389 w1390] -> w1376
                                frame Disabled {
                                n944 = local read item#-1() -> (w1389)
                                }
                                frame Enabled {
                                n945 = local read "heading error"() -> (w1393:dbl)
                                n946 = local read "POS init"() -> (w1391:bool)
                                n947 = Less?(x=w1393, y=0.1) -> (x < y?=w1392:bool)
                                n948 = Or(x=w1392, y=w1391) -> (x .or. y?=w1390:bool)
                                }
                                }
                                n949 = Index Array(array=w1373, index=3) -> (element=w1380:dbl)
                                n950 = global read "rio_Global.vi" "K"() -> (w1388:T12)
                                n951 = global read "rio_Global.vi" "H"() -> (w1387:T12)
                                n952 = global read "rio_Global.vi" "Pp"() -> (w1385:T12)
                                n953 = call-poly <vilib>:"Multiply.vi"("Real Matrix B"=w1387, "Real Matrix A"=w1388) -> ("A * B"=w1386:T12)
                                n954 = global read "rio_Global.vi" "Pp"() -> (w1383:T12)
                                n955 = call-poly <vilib>:"Multiply.vi"("Real Matrix B"=w1385, "Real Matrix A"=w1386) -> ("A * B"=w1384:T12)
                                n956 = call-poly <vilib>:"Subtract.vi"("Real Matrix B"=w1384, "Real Matrix A"=w1383) -> ("A - B"=w1382:T12)
                                n957 = global write "rio_Global.vi" "P"(w1382) -> ()
                                n958 = case shown="True" w1376 {
                                tunnel: w1380 -> [w1438 w1445]
                                tunnel: [w1438 w1440] -> w1374
                                frame False {
                                }
                                frame True {
                                n959 = global read "rio_Global.vi" "K"() -> (w1444:T12)
                                n960 = Index Array(array=w1444, index (row)=3, index (col)=2 ("disabled index (col)")) -> (element=w1441:dbl)
                                n961 = local read "h_gps"() -> (w1439:dbl)
                                n962 = call "headingweightsum2.vi"("a"=w1441, "h2"=w1439, "h1"=w1445) -> ("a*h2+(1-a)*h1"=w1440:dbl)  [unwired: 8 in]
                                }
                                }
                                n963 = case shown="True" w1375 {
                                tunnel: w1373 -> [w1414 w1426]
                                tunnel: [w1414 w1425] -> w1379
                                tunnel: w1374 -> [_ w1415]
                                frame False {
                                }
                                frame True {
                                n964 = disable-structure shown="Enabled" {
                                disable-tunnel: [w1436 w1437] -> w1416
                                disable-tunnel: w1415 -> [_ w1437]
                                frame Disabled {
                                n965 = local read item#-1() -> (w1436)
                                }
                                frame Enabled {
                                }
                                }
                                n966 = local read "pos_gps"() -> (w1420:dbl[])
                                n967 = call-poly <vilib>:"Array To Matrix.vi"("Real 1D Array"=w1426) -> ("Real Matrix (Column Vector)"=w1430:T12)
                                n968 = Array Subset(array=w1420, index=2, length=2) -> (w1421:dbl[])
                                n969 = Build Array (concatenate)(w1421, w1416) -> (w1417:dbl[])
                                n970 = global read "rio_Global.vi" "H"() -> (w1435:T12)
                                n971 = call-poly <vilib>:"Multiply.vi"("Real Matrix B"=w1430, "Real Matrix A"=w1435) -> ("A * B"=w1434:T12)
                                n972 = call-poly <vilib>:"Array To Matrix.vi"("Real 1D Array"=w1417) -> ("Real Matrix (Column Vector)"=w1433:T12)
                                n973 = call-poly <vilib>:"Subtract.vi"("Real Matrix B"=w1434, "Real Matrix A"=w1433) -> ("A - B"=w1431:T12)
                                n974 = global read "rio_Global.vi" "K"() -> (w1432:T12)
                                n975 = call-poly <vilib>:"Multiply.vi"("Real Matrix B"=w1431, "Real Matrix A"=w1432) -> ("A * B"=w1424:T12)
                                n976 = call-poly <vilib>:"Multiply.vi"("Real Matrix A"=w1424, "Real Scalar c"=0.25) -> ("c * A"=w1422:T12)
                                n977 = call-poly <vilib>:"Add.vi"("Real Matrix B"=w1430, "Real Matrix A"=w1422) -> ("A + B"=w1429:T12)
                                n978 = call-poly <vilib>:"Matrix To Array.vi"("Real Matrix"=w1429) -> ("Real 2D Array"=w1428:dbl[][])
                                n979 = Index Array(array=w1428, index (col)=0 ("disabled index (col)")) -> (element=w1425:dbl[])  [unwired: 1 in]
                                }
                                }
                                n980 = Replace Array Subset(array=w1379, new element=w1374, index=3) -> (w1377:dbl[])
                              }
                            }
                          }
                        }
                      }
                    }
                  }
                }
              }
            }
          }
          frame #2 {
            n981 = local read "h_gps"() -> (w1451:dbl)
            n982 = local read "dt"() -> (w1448:dbl)
            n983 = Index Array(array=w1462, index=3) -> (element=w1455:dbl)
            n984 = Array Subset(array=w1462, index=0, length=2) -> (→"pos":dbl[])
            n985 = Greater Than 0?(x=w1448) -> (x > 0?=w1447:bool)
            n986 = call "angleconv.vi"("rad"=w1455) -> ("deg"=→"Heading":dbl)  [unwired: 9 in, 1 out]
            n987 = Greater?(x=1.0, y=w1448) -> (0:w1450:bool)
            n988 = call "headingoperater.vi"("h1"=0.0, "h2"=w1451) -> ("h2+h1"=w1452:dbl)  [unwired: 8 in, 1 out]
            n989 = call "angleconv.vi"("rad"=w1452) -> ("deg"=→"H_GPS":dbl)  [unwired: 9 in, 1 out]
            n990 = Compound Arithmetic op=AND(w1450, w1447) -> (w1446:bool)
            n991 = case shown="True" w1446 {
              tunnel: w1462 -> [_ w1463]
              frame False {
              }
              frame True {
                n992 = flat-sequence {
                  tunnel: w1463 -> [w1487]
                  frame #0 {
                    n993 = Get Date/Time In Seconds() -> (seconds since 1Jan1904=w1478:timestamp)
                    n994 = To Double Precision Float(number=w1478) -> (double precision float=w1472:dbl)
                    n995 = global read "rio_Global.vi" "LCM_POS_T"() -> (w1486:T13)
                    n996 = local read "POS init"() -> (w1468:bool)
                    n997 = Unbundle By Name(w1486) -> ("hash"=w1483:i64)
                    n998 = local read "dt"() -> (w1467:dbl)
                    n999 = Multiply(x=w1472, y=1000000.0) -> (x*y=w1470:dbl)
                    n1000 = Array To Cluster(array=w1487) -> (cluster=w1485:T14)
                    n1001 = Select(t=0.0, s=w1468, f=w1467) -> (s? t:f=w1465:dbl)
                    n1002 = call "hash.vi"("input"=w1483) -> ("output"=w1482:i64)  [unwired: 10 in]
                    n1003 = To Quad Integer(1:w1470) -> (0:w1469:i64)
                    n1004 = Unbundle(w1485) -> ("Real 2D Array[0]"=w1477:dbl, "Real 2D Array[1]"=w1476:dbl, "Real 2D Array[2]"=w1475:dbl, "Real 2D Array[3]"=w1474:dbl, "Real 2D Array[4]"=w1473:dbl)
                    n1005 = Bundle(cluster=w1486, "hash"=w1482, "sys time"=w1469, "dt"=w1465, "x"=w1477, "y"=w1476, "speed"=w1475, "heading"=w1474, "yaw_rate"=w1473) -> (w1464:T13)
                    n1006 = Flatten To String(anything=w1464, prepend array or string size? (T)=FALSE) -> (data string=w1480:string)  [unwired: 2 in, 2 out]
                    n1007 = global read "rio_Global.vi" "LCM"() -> (w1479:T3)
                    n1008 = call "LCM_send.vi"("DATA"=w1480, "ID"="POS_T", "LCM"=w1479) -> ()  [unwired: 6 in, 3 out]
                  }
                }
              }
            }
          }
        }
      }
    }
  }
